vi "app - monitor RUS scan.vi"(10 "normalize phase":bool) -> ()   [LabVIEW 2015]
uses:
  complex region.ctl
  lorentzian.ctl
  circle corners.ctl
  cursor winow.ctl
  scale - offset gauge.ctl
  <vilib>/event_ctls.llb/eventvkey.ctl
  peak -- parameters -- complex fit.ctl
  wavepacket.ctl
  filter method control.ctl
  parameters -- scan monitor control.ctl
  monitor state.ctl
  peak monitor ctl - V2.ctl
  interpolation state - real.ctl
  countdown control.ctl
  cursor window action.ctl
  plot refs -- filter related.ctl
  monitor action.ctl
  read scan file control.ctl
  ctl -- name dispatcher -- action.ctl
  Q -- check range -- i -- real - window.vi
  array -- find interval - real.vi
  next chunk - read-write freq PID file - atomic actions .vi
  Q -- check range -- i -- integer.vi
  aggregator - vi - real - atomic.vi
  switch - C.vi
  acquire cursor window data.vi
  filter - complex - four.vi
  peak -- PM find lorenzian - V2.vi
  Q - not nan -- real.vi
  array -- find index - real.vi
  array -- interpolate -- i.vi
  Q - not nan -- integer.vi
  linear interpolation - real.vi
  tale of three indices.vi
  filter -- window span logic.vi
  linear interp iiii- complex - z-omega - divide.vi
  linear interpolation iiii- complex.vi
  containing bix.vi
  peak -- guess at omega -- dzdomega.vi
  command stack.vi
  tale of three indices -- check state.vi
  linear interp iiii- complex - z-omega.vi
  line -- complex.vi
  peak -- z center from mult phase points.vi
  peak -- estimate for lorentzian.vi
  peak -- fake phase around center.vi
  peak -- get weights.vi
  peak -- four corner circle transformation logic.vi
  peak - fit phase around center - V1.vi
  <vilib>/Analysis/baseanly.llb/A x B.vi
  <vilib>/Analysis/baseanly.llb/Complex A x B.vi
  circle center from three points.vi
  <vilib>/Utility/error.llb/Clear Errors.vi
  <vilib>/Utility/libraryn.llb/Check if File or Folder Exists.vi
  file -- read list of lines.vi
  parse -- find first line.vi
  parse -- get list of matches -- numbers.vi
  <vilib>/Utility/file.llb/Write To Spreadsheet File (string).vi
  <vilib>/gmath/function.llb/Binomial Coefficient.vi
  monitor -- write section files.vi
  <vilib>/Analysis/Matrix/Numeric/Conversions/Array To Matrix.vi
  <vilib>/Analysis/Matrix/Numeric/Conversions/Array To Matrix - RA2.vi
  <vilib>/Analysis/baseanly.llb/Inverse Matrix.vi
  <vilib>/Analysis/baseanly.llb/Real Inverse Matrix.vi
  array - generate range.vi
  peak -- fit function -- arctan.vi
  <vilib>/gmath/NumericalOptimization/Nonlinear Curve Fit.vi
  <vilib>/gmath/NumericalOptimization/Nonlinear Curve Fit LM.vi
  filter pipe - plot staff - more - V2.vi
panel:
  out "current resonance #":i32
  in  "overwriting !!":bool
  in  "current resonance #":i32
  in  "overwrite (d)":enum16{"DUMP", "WORK", ""}(ring)
  in  "Tab : monitor":enum32{"main", "EDIT"}(tab)=enum."EDIT"
  in  "scan monitor control":T1={"gamma acc. frac. - min "=0.3, "gamma acc frac.. - max"=3.0, "peak acc. fraction (af)"=5.0, "min peak acc. window (kHz)"=0.5, "use"=enum."fraction", "abs gamma min(kHz)"=0.005, "abs gamma max(kHz)"=5.0, "# points"=5, "gamma-factor (fa)"=5.0, "interpolate"=enum."line", "init"=TRUE, "Unique strike parameters"=TRUE, "max peak acc. window (kHz)"=10.0, "spacing factor"=1.5, "iterate #"=1, "overwrite ctl?"=FALSE, "write _m files?"=FALSE, "max slope (kHz/sweep)"=0.5, "funnel state"=enum."funnel open"}
  in  "monitor state":T2={"header - gamma"=[], "header - frequency"=[], "# of peaks"=32, "peaks OK"=FALSE}
  in  "autopilot":enum32{"on", "off"}(tab)=enum."off"
  in  "timer \"v\"":dbl(slide)=4.22200000169687 min=-2147482748.0000002 max=2129711151.0 step=0.01 scale=0.0..5.0 scale format="%#3_3f"
  in  "timer  \"update\"":dbl(slide)=9.242000002413988 min=-2147482714.9999983 max=2129711151.0 step=0.010000000000000002 scale=0.0..10.0 scale format="%#3_3f"
  in  "Temperature (K)":dbl=201.512
  in  "Magn Field (T)":dbl
  in  "Array of states":T3[](array[typedef])=[{"delta"=-0.0016575432837271364, "gamma"=0.76553, "exp"=652.9113, "found?"=TRUE, "found"=652.9096424567163, "gamma found"=0.7013829844109373, "init linear"=FALSE, "interpolate"=enum."line", "gamma-factor"=5.0, "slope"=-0.0044851701449078974, "update freq?"=TRUE, "update gamma?"=TRUE, "acc factor"=5.0, "linear interpolation state"={"requested size"=5, "Array"=[652.9241022479541, 652.9241022479541, 652.9081701289798, 652.9081701289798, 652.9096424567163], "actual number of elements"=5}, "ind"=0.0, "gamma ratio"=0.9162057455761854, "gamma off limit?"=FALSE, "freq off limit?"=FALSE}, {"delta"=0.003759118773814407, "gamma"=0.17466, "exp"=1036.47326, "found?"=TRUE, "found"=1036.4770191187738, "gamma found"=0.18203135700796666, "init linear"=FALSE, "interpolate"=enum."line", "gamma-factor"=5.0, "slope"=-0.0007907161774346605, "update freq?"=TRUE, "update gamma?"=TRUE, "acc factor"=5.0, "linear interpolation state"={"requested size"=5, "Array"=[1036.4789192628243, 1036.4789192628243, 1036.4748123891509, 1036.4748123891509, 1036.4770191187738], "actual number of elements"=5}, "ind"=1.0, "gamma ratio"=1.042204036459216, "gamma off limit?"=FALSE, "freq off limit?"=FALSE}, {"delta"=0.0049091040252733364, "gamma"=0.2876, "exp"=1456.4571, "found?"=TRUE, "found"=1456.4620091040254, "gamma found"=0.29018960202050387, "init linear"=FALSE, "interpolate"=enum."line", "gamma-factor"=5.0, "slope"=0.0005201884449343197, "update freq?"=TRUE, "update gamma?"=TRUE, "acc factor"=5.0, "linear interpolation state"={"requested size"=5, "Array"=[1456.4592147196108, 1456.4592147196108, 1456.4588278352328, 1456.4588278352328, 1456.4620091040254], "actual number of elements"=5}, "ind"=2.0, "gamma ratio"=1.0090041794871483, "gamma off limit?"=FALSE, "freq off limit?"=FALSE}, {"delta"=0.0007394967815343989, "gamma"=0.09637, "exp"=1508.93353, "found?"=TRUE, "found"=1508.9342694967816, "gamma found"=0.09651911838128847, "init linear"=FALSE, "interpolate"=enum."line", "gamma-factor"=5.0, "slope"=-0.00010129910398973152, "update freq?"=TRUE, "update gamma?"=TRUE, "acc factor"=5.0, "linear interpolation state"={"requested size"=5, "Array"=[1508.934330293854, 1508.934330293854, 1508.9334388969608, 1508.9334388969608, 1508.9342694967816], "actual number of elements"=5}, "ind"=3.0, "gamma ratio"=1.0015473527164935, "gamma off limit?"=FALSE, "freq off limit?"=FALSE}, {"delta"=-0.029278381005497067, "gamma"=0.50061, "exp"=1568.62295, "found?"=TRUE, "found"=1568.5936716189944, "gamma found"=0.29241762919205017, "init linear"=FALSE, "interpolate"=enum."line", "gamma-factor"=5.0, "slope"=0.002435031997738406, "update freq?"=TRUE, "update gamma?"=TRUE, "acc factor"=5.0, "linear interpolation state"={"requested size"=5, "Array"=[1568.5938152073131, 1568.5938152073131, 1568.618452703927, 1568.618452703927, 1568.5936716189944], "actual number of elements"=5}, "ind"=4.0, "gamma ratio"=0.5841226287769924, "gamma off limit?"=FALSE, "freq off limit?"=FALSE}, {"delta"=0.0026202347487469524, "gamma"=0.0806, "exp"=1635.60553, "found?"=TRUE, "found"=1635.6081502347488, "gamma found"=0.08233227541925552, "init linear"=FALSE, "interpolate"=enum."line", "gamma-factor"=5.0, "slope"=-0.0002922362121171318, "update freq?"=TRUE, "update gamma?"=TRUE, "acc factor"=5.0, "linear interpolation state"={"requested size"=5, "Array"=[1635.6087113801916, 1635.6087113801916, 1635.6069113089588, 1635.6069113089588, 1635.6081502347488], "actual number of elements"=5}, "ind"=5.0, "gamma ratio"=1.0214922508592494, "gamma off limit?"=FALSE, "freq off limit?"=FALSE}, {"delta"=-0.002563017279953783, "gamma"=0.23948, "exp"=1764.33943, "found?"=TRUE, "found"=1764.33686698272, "gamma found"=0.24236340731954384, "init linear"=FALSE, "interpolate"=enum."line", "gamma-factor"=5.0, "slope"=-0.0006999494679621421, "update freq?"=TRUE, "update gamma?"=TRUE, "acc factor"=5.0, "linear interpolation state"={"requested size"=5, "Array"=[1764.3399842040806, 1764.3399842040806, 1764.339219152121, 1764.339219152121, 1764.33686698272], "actual number of elements"=5}, "ind"=6.0, "gamma ratio"=1.012040284447736, "gamma off limit?"=FALSE, "freq off limit?"=FALSE}, {"delta"=0.0013207520305513754, "gamma"=0.09629, "exp"=2205.10687, "found?"=TRUE, "found"=2205.1081907520306, "gamma found"=0.0924387831546914, "init linear"=FALSE, "interpolate"=enum."line", "gamma-factor"=5.0, "slope"=-7.088923128321767e-05, "update freq?"=TRUE, "update gamma?"=TRUE, "acc factor"=5.0, "linear interpolation state"={"requested size"=5, "Array"=[2205.108115975172, 2205.108115975172, 2205.1072575291464, 2205.1072575291464, 2205.1081907520306], "actual number of elements"=5}, "ind"=7.0, "gamma ratio"=0.9600039791742797, "gamma off limit?"=FALSE, "freq off limit?"=FALSE}, {"delta"=0.003409232488138514, "gamma"=0.15471, "exp"=2247.57115, "found?"=TRUE, "found"=2247.5745592324884, "gamma found"=0.1527741784741036, "init linear"=FALSE, "interpolate"=enum."line", "gamma-factor"=5.0, "slope"=-0.0009672962635522708, "update freq?"=TRUE, "update gamma?"=TRUE, "acc factor"=5.0, "linear interpolation state"={"requested size"=5, "Array"=[2247.5776758034717, 2247.5776758034717, 2247.574235982803, 2247.574235982803, 2247.5745592324884], "actual number of elements"=5}, "ind"=8.0, "gamma ratio"=0.9874874182283214, "gamma off limit?"=FALSE, "freq off limit?"=FALSE}, {"delta"=-0.008548894449631916, "gamma"=0.16479, "exp"=2285.77663, "found?"=TRUE, "found"=2285.76808110555, "gamma found"=0.1267187147828005, "init linear"=FALSE, "interpolate"=enum."line", "gamma-factor"=5.0, "slope"=-0.0016395337344147264, "update freq?"=TRUE, "update gamma?"=TRUE, "acc factor"=5.0, "linear interpolation state"={"requested size"=5, "Array"=[2285.7766292086317, 2285.7766292086317, 2285.77733007745, 2285.77733007745, 2285.76808110555], "actual number of elements"=5}, "ind"=9.0, "gamma ratio"=0.7689709010425421, "gamma off limit?"=FALSE, "freq off limit?"=FALSE}, {"delta"=0.0004447395758688799, "gamma"=0.21964, "exp"=2405.10472, "found?"=TRUE, "found"=2405.1051647395757, "gamma found"=0.22044726667002684, "init linear"=FALSE, "interpolate"=enum."line", "gamma-factor"=5.0, "slope"=-0.0008384914183989168, "update freq?"=TRUE, "update gamma?"=TRUE, "acc factor"=5.0, "linear interpolation state"={"requested size"=5, "Array"=[2405.1081612139637, 2405.1081612139637, 2405.10576924856, 2405.10576924856, 2405.1051647395757], "actual number of elements"=5}, "ind"=10.0, "gamma ratio"=1.0036754082590915, "gamma off limit?"=FALSE, "freq off limit?"=FALSE}, {"delta"=0.0003001280488206248, "gamma"=0.22537, "exp"=2483.53635, "found?"=TRUE, "found"=2483.5366501280487, "gamma found"=0.2213622002178064, "init linear"=FALSE, "interpolate"=enum."line", "gamma-factor"=5.0, "slope"=-5.884840269573033e-05, "update freq?"=TRUE, "update gamma?"=TRUE, "acc factor"=5.0, "linear interpolation state"={"requested size"=5, "Array"=[2483.536882570466, 2483.536882570466, 2483.5367589712696, 2483.5367589712696, 2483.5366501280487], "actual number of elements"=5}, "ind"=11.0, "gamma ratio"=0.9822168000080153, "gamma off limit?"=FALSE, "freq off limit?"=FALSE}, {"delta"=-0.00047377254441016703, "gamma"=0.1374, "exp"=2613.48596, "found?"=TRUE, "found"=2613.4854862274556, "gamma found"=0.13919976502630776, "init linear"=FALSE, "interpolate"=enum."line", "gamma-factor"=5.0, "slope"=-0.0004374731567804702, "update freq?"=TRUE, "update gamma?"=TRUE, "acc factor"=5.0, "linear interpolation state"={"requested size"=5, "Array"=[2613.4871697330486, 2613.4871697330486, 2613.4861620126653, 2613.4861620126653, 2613.4854862274556], "actual number of elements"=5}, "ind"=12.0, "gamma ratio"=1.0130987265379023, "gamma off limit?"=FALSE, "freq off limit?"=FALSE}, {"delta"=-0.0014333203166643216, "gamma"=0.23275, "exp"=2775.83282, "found?"=TRUE, "found"=2775.8313866796834, "gamma found"=0.2800873248387451, "init linear"=FALSE, "interpolate"=enum."line", "gamma-factor"=5.0, "slope"=9.053546469658613e-05, "update freq?"=TRUE, "update gamma?"=TRUE, "acc factor"=5.0, "linear interpolation state"={"requested size"=5, "Array"=[2775.8316113301, 2775.8316113301, 2775.8329659855785, 2775.8329659855785, 2775.8313866796834], "actual number of elements"=5}, "ind"=13.0, "gamma ratio"=1.2033827060740927, "gamma off limit?"=FALSE, "freq off limit?"=FALSE}, {"delta"=0.001513914386578108, "gamma"=0.0716, "exp"=2886.62499, "found?"=TRUE, "found"=2886.6265039143864, "gamma found"=0.07112662438840253, "init linear"=FALSE, "interpolate"=enum."line", "gamma-factor"=5.0, "slope"=-0.0006266225839499384, "update freq?"=TRUE, "update gamma?"=TRUE, "acc factor"=5.0, "linear interpolation state"={"requested size"=5, "Array"=[2886.628416499212, 2886.628416499212, 2886.6259754430316, 2886.6259754430316, 2886.6265039143864], "actual number of elements"=5}, "ind"=14.0, "gamma ratio"=0.9933886087765718, "gamma off limit?"=FALSE, "freq off limit?"=FALSE}, {"delta"=0.006262894615701953, "gamma"=0.14682, "exp"=2925.52376, "found?"=TRUE, "found"=2925.5300228946157, "gamma found"=0.14212049264176846, "init linear"=FALSE, "interpolate"=enum."line", "gamma-factor"=5.0, "slope"=-0.0013607249583583326, "update freq?"=TRUE, "update gamma?"=TRUE, "acc factor"=5.0, "linear interpolation state"={"requested size"=5, "Array"=[2925.5337999193525, 2925.5337999193525, 2925.5277467192377, 2925.5277467192377, 2925.5300228946157], "actual number of elements"=5}, "ind"=15.0, "gamma ratio"=0.9679913679455691, "gamma off limit?"=FALSE, "freq off limit?"=FALSE}, {"delta"=0.0008407358172917156, "gamma"=0.05724, "exp"=2968.74884, "found?"=TRUE, "found"=2968.7496807358175, "gamma found"=0.056604877858379594, "init linear"=FALSE, "interpolate"=enum."line", "gamma-factor"=5.0, "slope"=6.453693960793316e-05, "update freq?"=TRUE, "update gamma?"=TRUE, "acc factor"=5.0, "linear interpolation state"={"requested size"=5, "Array"=[2968.7492258726284, 2968.7492258726284, 2968.7489615156423, 2968.7489615156423, 2968.7496807358175], "actual number of elements"=5}, "ind"=16.0, "gamma ratio"=0.9889042253385674, "gamma off limit?"=FALSE, "freq off limit?"=FALSE}, {"delta"=0.0004893467435067578, "gamma"=0.18507, "exp"=3117.27562, "found?"=TRUE, "found"=3117.2761093467434, "gamma found"=0.18508310581473786, "init linear"=FALSE, "interpolate"=enum."line", "gamma-factor"=5.0, "slope"=-0.000674382079159841, "update freq?"=TRUE, "update gamma?"=TRUE, "acc factor"=5.0, "linear interpolation state"={"requested size"=5, "Array"=[3117.278479994366, 3117.278479994366, 3117.27647746882, 3117.27647746882, 3117.2761093467434], "actual number of elements"=5}, "ind"=17.0, "gamma ratio"=1.0000708154467923, "gamma off limit?"=FALSE, "freq off limit?"=FALSE}, {"delta"=0.0009432243264200224, "gamma"=0.11467, "exp"=3141.4319, "found?"=TRUE, "found"=3141.4328432243265, "gamma found"=0.11506466086057514, "init linear"=FALSE, "interpolate"=enum."line", "gamma-factor"=5.0, "slope"=-0.0002722086093854159, "update freq?"=TRUE, "update gamma?"=TRUE, "acc factor"=5.0, "linear interpolation state"={"requested size"=5, "Array"=[3141.4337316093643, 3141.4337316093643, 3141.432786293347, 3141.432786293347, 3141.4328432243265], "actual number of elements"=5}, "ind"=18.0, "gamma ratio"=1.0034417097808943, "gamma off limit?"=FALSE, "freq off limit?"=FALSE}, {"delta"=0.006890674223541282, "gamma"=0.19401, "exp"=3268.65403, "found?"=TRUE, "found"=3268.6609206742237, "gamma found"=0.1947000973954296, "init linear"=FALSE, "interpolate"=enum."line", "gamma-factor"=5.0, "slope"=0.001370561413350515, "update freq?"=TRUE, "update gamma?"=TRUE, "acc factor"=5.0, "linear interpolation state"={"requested size"=5, "Array"=[3268.654487682439, 3268.654487682439, 3268.6553273130035, 3268.6553273130035, 3268.6609206742237], "actual number of elements"=5}, "ind"=19.0, "gamma ratio"=1.0035570197176928, "gamma off limit?"=FALSE, "freq off limit?"=FALSE}, {"delta"=-0.00036122355459156097, "gamma"=0.09375, "exp"=3447.74234, "found?"=TRUE, "found"=3447.741978776445, "gamma found"=0.09343849466512388, "init linear"=FALSE, "interpolate"=enum."line", "gamma-factor"=5.0, "slope"=-0.0002539216459263116, "update freq?"=TRUE, "update gamma?"=TRUE, "acc factor"=5.0, "linear interpolation state"={"requested size"=5, "Array"=[3447.7428802682552, 3447.7428802682552, 3447.742144035429, 3447.742144035429, 3447.741978776445], "actual number of elements"=5}, "ind"=20.0, "gamma ratio"=0.9966772764279881, "gamma off limit?"=FALSE, "freq off limit?"=FALSE}, {"delta"=-3486.5123, "gamma"=0.01485, "exp"=3486.5123, "found?"=FALSE, "found"=0.0, "gamma found"=0.0, "init linear"=TRUE, "interpolate"=enum."line", "gamma-factor"=5.0, "slope"=0.0, "update freq?"=FALSE, "update gamma?"=FALSE, "acc factor"=5.0, "linear interpolation state"={"requested size"=5, "Array"=[0.0, 0.0, 0.0, 0.0, 3486.5122984940626], "actual number of elements"=1}, "ind"=21.0, "gamma ratio"=0.0, "gamma off limit?"=TRUE, "freq off limit?"=TRUE}, {"delta"=0.005188108485072007, "gamma"=0.2862, "exp"=3737.75053, "found?"=TRUE, "found"=3737.755718108485, "gamma found"=0.25947921890028686, "init linear"=FALSE, "interpolate"=enum."line", "gamma-factor"=5.0, "slope"=-0.0006564744841307402, "update freq?"=TRUE, "update gamma?"=TRUE, "acc factor"=5.0, "linear interpolation state"={"requested size"=5, "Array"=[3737.7568178710067, 3737.7568178710067, 3737.752452651206, 3737.752452651206, 3737.755718108485], "actual number of elements"=5}, "ind"=22.0, "gamma ratio"=0.9066359849765439, "gamma off limit?"=FALSE, "freq off limit?"=FALSE}, {"delta"=0.05791749378431632, "gamma"=0.1209, "exp"=3773.78708, "found?"=FALSE, "found"=3773.8449974937844, "gamma found"=0.0018969298658040622, "init linear"=FALSE, "interpolate"=enum."line", "gamma-factor"=7.0, "slope"=-0.027493364620750072, "update freq?"=TRUE, "update gamma?"=TRUE, "acc factor"=7.0, "linear interpolation state"={"requested size"=5, "Array"=[0.0, 3773.880271706499, 3773.8206547185614, 3773.825284977259, 3773.7870837381997], "actual number of elements"=4}, "ind"=23.0, "gamma ratio"=0.015690073331712674, "gamma off limit?"=TRUE, "freq off limit?"=FALSE}, {"delta"=0.0016448427732029813, "gamma"=0.14541, "exp"=4176.53307, "found?"=TRUE, "found"=4176.534714842774, "gamma found"=0.14055145401454877, "init linear"=FALSE, "interpolate"=enum."line", "gamma-factor"=5.0, "slope"=0.001082140458165668, "update freq?"=TRUE, "update gamma?"=TRUE, "acc factor"=5.0, "linear interpolation state"={"requested size"=5, "Array"=[4176.530918624351, 4176.530918624351, 4176.534147592093, 4176.534147592093, 4176.534714842774], "actual number of elements"=5}, "ind"=24.0, "gamma ratio"=0.9665872636995307, "gamma off limit?"=FALSE, "freq off limit?"=FALSE}, {"delta"=0.006093070963288483, "gamma"=0.07631, "exp"=4238.40966, "found?"=TRUE, "found"=4238.415753070964, "gamma found"=0.07370934433890397, "init linear"=FALSE, "interpolate"=enum."line", "gamma-factor"=5.0, "slope"=-0.0001927513594273478, "update freq?"=TRUE, "update gamma?"=TRUE, "acc factor"=5.0, "linear interpolation state"={"requested size"=5, "Array"=[4238.415194475135, 4238.415194475135, 4238.412149769886, 4238.412149769886, 4238.415753070964], "actual number of elements"=5}, "ind"=25.0, "gamma ratio"=0.9659198576713925, "gamma off limit?"=FALSE, "freq off limit?"=FALSE}, {"delta"=0.0014712240090375417, "gamma"=0.10797, "exp"=4931.57573, "found?"=TRUE, "found"=4931.577201224009, "gamma found"=0.1106825599113035, "init linear"=FALSE, "interpolate"=enum."line", "gamma-factor"=5.0, "slope"=0.0010064907773630694, "update freq?"=TRUE, "update gamma?"=TRUE, "acc factor"=5.0, "linear interpolation state"={"requested size"=5, "Array"=[4931.573629158262, 4931.573629158262, 4931.5765499345425, 4931.5765499345425, 4931.577201224009], "actual number of elements"=5}, "ind"=26.0, "gamma ratio"=1.0251232741622998, "gamma off limit?"=FALSE, "freq off limit?"=FALSE}, {"delta"=0.01094153662052122, "gamma"=0.05188, "exp"=5475.82656, "found?"=TRUE, "found"=5475.837501536621, "gamma found"=0.11863591544266465, "init linear"=FALSE, "interpolate"=enum."line", "gamma-factor"=8.0, "slope"=0.0012847163761034609, "update freq?"=TRUE, "update gamma?"=TRUE, "acc factor"=8.0, "linear interpolation state"={"requested size"=5, "Array"=[5475.831455900791, 5475.831455900791, 5475.832211792886, 5475.832211792886, 5475.837501536621], "actual number of elements"=5}, "ind"=27.0, "gamma ratio"=2.2867369977383314, "gamma off limit?"=FALSE, "freq off limit?"=FALSE}, {"delta"=-5768.35916, "gamma"=0.005, "exp"=5768.35916, "found?"=FALSE, "found"=0.0, "gamma found"=0.0, "init linear"=TRUE, "interpolate"=enum."line", "gamma-factor"=5.0, "slope"=0.0, "update freq?"=FALSE, "update gamma?"=FALSE, "acc factor"=5.0, "linear interpolation state"={"requested size"=5, "Array"=[0.0, 0.0, 0.0, 0.0, 5768.359158074293], "actual number of elements"=1}, "ind"=28.0, "gamma ratio"=0.0, "gamma off limit?"=TRUE, "freq off limit?"=TRUE}, {"delta"=18.256138418231785, "gamma"=0.02905, "exp"=6148.70194, "found?"=FALSE, "found"=6166.958078418232, "gamma found"=4.5314912463139816e-05, "init linear"=TRUE, "interpolate"=enum."line", "gamma-factor"=5.0, "slope"=0.0, "update freq?"=FALSE, "update gamma?"=FALSE, "acc factor"=5.0, "linear interpolation state"={"requested size"=5, "Array"=[0.0, 0.0, 0.0, 0.0, 6148.701943422434], "actual number of elements"=1}, "ind"=29.0, "gamma ratio"=0.001559893716459202, "gamma off limit?"=TRUE, "freq off limit?"=TRUE}, {"delta"=0.004358224254247034, "gamma"=0.0424, "exp"=5751.24344, "found?"=TRUE, "found"=5751.247798224254, "gamma found"=0.0686871247901866, "init linear"=TRUE, "interpolate"=enum."line", "gamma-factor"=7.0, "slope"=0.0, "update freq?"=FALSE, "update gamma?"=FALSE, "acc factor"=7.0, "linear interpolation state"={"requested size"=5, "Array"=[0.0, 0.0, 0.0, 0.0, 5751.24344], "actual number of elements"=1}, "ind"=30.0, "gamma ratio"=1.619979358259118, "gamma off limit?"=FALSE, "freq off limit?"=FALSE}, {"delta"=0.02459476473813993, "gamma"=0.14229, "exp"=6300.95565, "found?"=TRUE, "found"=6300.980244764738, "gamma found"=0.1593322314931949, "init linear"=FALSE, "interpolate"=enum."line", "gamma-factor"=7.0, "slope"=0.001076212803600356, "update freq?"=TRUE, "update gamma?"=TRUE, "acc factor"=7.0, "linear interpolation state"={"requested size"=5, "Array"=[6300.9711810739645, 6300.9711810739645, 6300.963815820454, 6300.963815820454, 6300.980244764738], "actual number of elements"=5}, "ind"=31.0, "gamma ratio"=1.1197711117660756, "gamma off limit?"=FALSE, "freq off limit?"=FALSE}]
  in  "dump/work NEW (\"n\")":enum16{"DUMP", "WORK", ""}(ring)
  in  "NEW freq":dbl[](array[numeric])=[652.901381931682, 1036.4745243360126, 1456.4611794080774, 1508.93365767837, 1568.6109465842878, 1635.607002413974, 1764.33695489062, 2205.1075748844396, 2247.5727746722177, 2285.770281334339, 2405.104089658669, 2483.536610097096, 2613.485117524306, 2775.8323798686024, 2886.625177692022, 2925.5265410594843, 2968.74940471329, 3117.275181708386, 3141.432359180121, 3268.6602218172616, 3447.7416437118245, 3486.5122984940626, 3737.7528824071287, 3773.7595903735782, 4176.536215876507, 4238.4135100581225, 4931.5785313542565, 5475.8368215339215, 5768.359158074293, 6148.701943422434, 5751.24344, 6300.973276349126]
  in  "NEW gamma":dbl[](array[numeric])=[0.7013829844109373, 0.18203135700796666, 0.29018960202050387, 0.09651911838128847, 0.29241762919205017, 0.08233227541925552, 0.24236340731954384, 0.0924387831546914, 0.1527741784741036, 0.1267187147828005, 0.22044726667002684, 0.2213622002178064, 0.13919976502630776, 0.2800873248387451, 0.07112662438840253, 0.14212049264176846, 0.056604877858379594, 0.18508310581473786, 0.11506466086057514, 0.1947000973954296, 0.09343849466512388, 0.01485, 0.25947921890028686, 0.1209, 0.14055145401454877, 0.07370934433890397, 0.1106825599113035, 0.11863591544266465, 0.005, 0.02905, 0.0424, 0.1593322314931949]
  in  "OLD gamma":dbl[](array[numeric])
  in  "OLD freq":dbl[](array[numeric])
  out "cp lorentzian":T5={"Amplitude"=0.017781649209978104, "omega(0)"=653.3752688609701, "Gamma"=64.36082364251368, "phase"=2.362044339201428, "Q"=10.151754310822424, "Norm  Ampl"=nan, "z (inf)"=0.02262747381101565+0.008890453242250202i, "4corners"={"z (-pi/2)"=0.022625188172095752+0.009281166377616138i, "z(inf)"=0.02262747381101565+0.008890453242250202i, "z (pi/2)"=0.023018186946381587+0.008892738881170098i, "z center"=0.02282168755923867+0.009086952629393118i, "z(0)"=0.02301590130746169+0.009283452016536034i, "radius"=0.0002762806347654071}} {"z (inf)" format="%#9_9f"; "Q" format="%#9_9f"; "phase" format="%#9_9f"; "Gamma" format="%#9_9f"; "omega(0)" format="%#9_9f"}
  out "index":i32[](array[numeric])=[0, 1, 2, 3, 4, 5, 6, 7, 8, 9, 10, 11, 12, 13, 14, 15, 16, 17, 18, 19, 20, 21, 22, 23, 24, 25, 26, 27, 28, 29, 30, 31, 32, 33, 34, 35, 36, 37, 38, 39, 40, 41, 42, 43, 44, 45, 46, 47, 48, 49, 50, 51, 52, 53, 54, 55, 56, 57, 58, 59, 60, 61, 62, 63, 64, 65, 66, 67, 68, 69, 70, 71, 72, 73, 74, 75, 76, 77, 78, 79, 80, 81, 82, 83, 84, 85, 86, 87, 88, 89, 90, 91, 92, 93, 94, 95, 96, 97, 98, 99]
  in  "Tab : everything":T7(tab)
  in  "Tab :  Fit controls":enum32{"complex plane", "complex plane 2"}(tab)
  in  "Plot: fragment - filter":cluster{dbl[], dbl[]}[](graph)
  in  "scale gauge: Plot: complex plane - filter":dbl(slide)=0.00996 min=0.0 max=0.3 step=1e-05 scale=0.0001..0.3 scale format="%#_2g"
  in  "Plot: complex plane - filter":cluster{dbl[], dbl[]}[](graph)=[{array[252 elements], array[252 elements]}, {array[252 elements], array[252 elements]}, {[0.02330588676949013, 0.023305318955812702, 0.023303617755681592, 0.02330078988295652, 0.02329684649795919, 0.023291803163428635, 0.02328567978310216, 0.023278500523164408, 0.023270293716874463, 0.023261091752747418, 0.023250930946731706, 0.023239851398886638, 0.023227896835125793, 0.02321511443465082, 0.023201554643756665, 0.023187270976743113, 0.02317231980471828, 0.023156760133127598, 0.023140653368886308, 0.02312406307803438, 0.023107054734870437, 0.023089695463554563, 0.023072053773199947, 0.023054199287498703, 0.023036202469948946, 0.02301813434576759, 0.023000066221586235, 0.02298206940403648, 0.022964214918335234, 0.02294657322798062, 0.022929213956664744, 0.0229122056135008, 0.022895615322648874, 0.022879508558407584, 0.022863948886816903, 0.02284899771479207, 0.022834714047778516, 0.02282115425688436, 0.02280837185640939, 0.022796417292648544, 0.022785337744803475, 0.022775176938787764, 0.022765974974660718, 0.022757768168370773, 0.022750588908433022, 0.022744465528106547, 0.02273942219357599, 0.022735478808578662, 0.02273265093585359, 0.02273094973572248, 0.022730381922045052, 0.02273094973572248, 0.02273265093585359, 0.022735478808578662, 0.02273942219357599, 0.022744465528106547, 0.022750588908433022, 0.022757768168370773, 0.022765974974660718, 0.022775176938787764, 0.022785337744803475, 0.022796417292648544, 0.02280837185640939, 0.02282115425688436, 0.022834714047778516, 0.02284899771479207, 0.022863948886816903, 0.022879508558407584, 0.022895615322648877, 0.0229122056135008, 0.022929213956664744, 0.02294657322798062, 0.022964214918335234, 0.02298206940403648, 0.023000066221586235, 0.02301813434576759, 0.023036202469948946, 0.023054199287498703, 0.023072053773199947, 0.023089695463554563, 0.023107054734870437, 0.02312406307803438, 0.023140653368886304, 0.023156760133127598, 0.02317231980471828, 0.023187270976743113, 0.023201554643756665, 0.02321511443465082, 0.023227896835125793, 0.023239851398886638, 0.023250930946731706, 0.023261091752747418, 0.023270293716874463, 0.023278500523164408, 0.02328567978310216, 0.023291803163428635, 0.02329684649795919, 0.02330078988295652, 0.023303617755681592, 0.023305318955812702], [0.009264160688823775, 0.009282228813005132, 0.009300225630554887, 0.009318080116256133, 0.009335721806610747, 0.00935308107792662, 0.009370089421090565, 0.00938667971194249, 0.009402786476183781, 0.00941834614777446, 0.009433297319799297, 0.00944758098681285, 0.009461140777707005, 0.009473923178181978, 0.00948587774194282, 0.009496957289787888, 0.009507118095803603, 0.009516320059930647, 0.009524526866220592, 0.009531706126158343, 0.009537829506484819, 0.009542872841015376, 0.009546816226012703, 0.009549644098737778, 0.009551345298868886, 0.009551913112546313, 0.009551345298868886, 0.009549644098737778, 0.009546816226012703, 0.009542872841015376, 0.009537829506484819, 0.009531706126158343, 0.009524526866220592, 0.009516320059930647, 0.009507118095803603, 0.009496957289787888, 0.00948587774194282, 0.009473923178181978, 0.009461140777707005, 0.00944758098681285, 0.009433297319799297, 0.00941834614777446, 0.009402786476183781, 0.00938667971194249, 0.009370089421090565, 0.00935308107792662, 0.009335721806610747, 0.009318080116256133, 0.009300225630554887, 0.009282228813005132, 0.009264160688823775, 0.009246092564642417, 0.009228095747092662, 0.009210241261391416, 0.009192599571036802, 0.00917524029972093, 0.009158231956556982, 0.00914164166570506, 0.009125534901463768, 0.009109975229873089, 0.009095024057848252, 0.009080740390834698, 0.009067180599940544, 0.00905439819946557, 0.00904244363570473, 0.00903136408785966, 0.009021203281843946, 0.009012001317716902, 0.009003794511426957, 0.008996615251489206, 0.00899049187116273, 0.008985448536632173, 0.008981505151634846, 0.008978677278909771, 0.008976976078778664, 0.008976408265101236, 0.008976976078778664, 0.008978677278909771, 0.008981505151634846, 0.008985448536632173, 0.00899049187116273, 0.008996615251489206, 0.009003794511426957, 0.009012001317716902, 0.009021203281843946, 0.00903136408785966, 0.00904244363570473, 0.00905439819946557, 0.009067180599940544, 0.009080740390834698, 0.009095024057848252, 0.009109975229873089, 0.009125534901463768, 0.00914164166570506, 0.009158231956556984, 0.00917524029972093, 0.009192599571036804, 0.009210241261391416, 0.009228095747092662, 0.009246092564642417]}, {[-7.134950150070041e-05, 3.845143540140428e-06, 3.702069766946953e-05], [0.0001830739588743243, -6.1760698272413095e-06, -3.90775167372244e-06]}, {[-3.448933898232793e-05, -3.695183869243852e-05, -3.941433840254912e-05, -4.1876838112659715e-05, -4.433933782277031e-05, -4.680183753288091e-05, -4.926433724299151e-05, -5.1726836953102105e-05, -5.41893366632127e-05, -5.66518363733233e-05, -5.911433608343389e-05, -6.157683579354449e-05, -6.403933550365509e-05, -6.65018352137657e-05, -6.896433492387628e-05, -7.142683463398687e-05, -7.388933434409748e-05, -7.635183405420808e-05, -7.881433376431867e-05, -8.127683347442926e-05], [3.604811685728011e-05, 3.82835879236857e-05, 4.051905899009129e-05, 4.275453005649688e-05, 4.499000112290247e-05, 4.722547218930806e-05, 4.9460943255713647e-05, 5.169641432211924e-05, 5.393188538852483e-05, 5.616735645493042e-05, 5.840282752133601e-05, 6.063829858774159e-05, 6.287376965414718e-05, 6.510924072055277e-05, 6.734471178695836e-05, 6.958018285336396e-05, 7.181565391976955e-05, 7.405112498617514e-05, 7.628659605258073e-05, 7.852206711898632e-05]}, {[3.845143540140428e-06, 8.708015624839466e-06, 1.3570887709538504e-05, 1.843375979423754e-05, 2.329663187893658e-05, 2.815950396363562e-05, 3.302237604833465e-05, 3.788524813303369e-05, 4.274812021773273e-05, 4.761099230243177e-05, 5.247386438713081e-05, 5.7336736471829845e-05, 6.219960855652888e-05, 6.706248064122792e-05, 7.192535272592696e-05, 7.6788224810626e-05, 8.165109689532504e-05, 8.651396898002407e-05, 9.137684106472312e-05, 9.623971314942215e-05], [-6.1760698272413095e-06, -6.1760698272413095e-06, -6.1760698272413095e-06, -6.1760698272413095e-06, -6.1760698272413095e-06, -6.1760698272413095e-06, -6.1760698272413095e-06, -6.1760698272413095e-06, -6.1760698272413095e-06, -6.1760698272413095e-06, -6.1760698272413095e-06, -6.1760698272413095e-06, -6.1760698272413095e-06, -6.1760698272413095e-06, -6.1760698272413095e-06, -6.1760698272413095e-06, -6.1760698272413095e-06, -6.1760698272413095e-06, -6.1760698272413095e-06, -6.1760698272413095e-06]}]
  out "Plot: dz/domega":cluster{"omega out":dbl[], dbl[]}(graph)
  out "Plot: win omega":T8(graph)
  out "Plot: phase":cluster{"omega out":dbl[], dbl[]}(graph)
  out "Plot: phase around center":cluster{dbl[], dbl[]}[](graph)
  out "Plot: fragment":cluster{dbl[], dbl[]}[](graph)
  out "Plot: complex plane":cluster{dbl[], dbl[]}[](graph)=[{array[252 elements], array[252 elements]}, {[0.023097968194004077, 0.023095789638677925, 0.023089288329818373, 0.023078566796949824, 0.023063794125050354, 0.02304520328798058, 0.023023087474346726, 0.022997795463741137, 0.02296972612627978, 0.022939322132182232, 0.02290706297059788, 0.02287345738777559, 0.02283903536383148, 0.02280433975464586, 0.02276991773070175, 0.02273631214787946, 0.022704052986295107, 0.022673648992197558, 0.022645579654736202, 0.022620287644130613, 0.02259817183049676, 0.022579580993426985, 0.022564808321527515, 0.022554086788658965, 0.022547585479799414, 0.022545406924473262, 0.022547585479799414, 0.022554086788658965, 0.022564808321527515, 0.022579580993426985, 0.02259817183049676, 0.022620287644130613, 0.022645579654736202, 0.022673648992197558, 0.022704052986295107, 0.02273631214787946, 0.02276991773070175, 0.02280433975464586, 0.02283903536383148, 0.02287345738777559, 0.02290706297059788, 0.022939322132182232, 0.02296972612627978, 0.022997795463741137, 0.023023087474346726, 0.02304520328798058, 0.023063794125050354, 0.023078566796949824, 0.023089288329818373, 0.023095789638677925], [0.009086952629393118, 0.009121579774719465, 0.009155660829278761, 0.009188658314481572, 0.009220051840274506, 0.009249346312002228, 0.009276079738345919, 0.009299830517202365, 0.009320224084600974, 0.009336938821801342, 0.00934971112741292, 0.009358339574546407, 0.009362688087436124, 0.009362688087436124, 0.009358339574546407, 0.00934971112741292, 0.009336938821801342, 0.009320224084600974, 0.009299830517202365, 0.009276079738345919, 0.009249346312002228, 0.009220051840274506, 0.009188658314481572, 0.009155660829278761, 0.009121579774719465, 0.009086952629393118, 0.009052325484066771, 0.009018244429507475, 0.008985246944304663, 0.008953853418511728, 0.008924558946784008, 0.008897825520440317, 0.00887407474158387, 0.008853681174185262, 0.008836966436984894, 0.008824194131373315, 0.008815565684239829, 0.008811217171350113, 0.008811217171350113, 0.008815565684239829, 0.008824194131373315, 0.008836966436984894, 0.008853681174185262, 0.008874074741583872, 0.008897825520440317, 0.008924558946784008, 0.00895385341851173, 0.008985246944304665, 0.009018244429507475, 0.009052325484066771]}, {[0.02262747381101565, 0.02264689518583795, 0.022666316560660253, 0.022685737935482557, 0.022705159310304857, 0.022724580685127158, 0.02274400205994946, 0.022763423434771765, 0.022782844809594065, 0.022802266184416366, 0.02282168755923867, 0.022841108934060973, 0.022860530308883274, 0.022879951683705574, 0.022899373058527878, 0.02291879443335018, 0.02293821580817248, 0.022957637182994782, 0.022977058557817086, 0.02299647993263939], [0.008890453242250202, 0.008910103180964494, 0.008929753119678785, 0.008949403058393077, 0.008969052997107369, 0.008988702935821661, 0.009008352874535951, 0.009028002813250243, 0.009047652751964536, 0.009067302690678826, 0.009086952629393118, 0.00910660256810741, 0.0091262525068217, 0.009145902445535993, 0.009165552384250285, 0.009185202322964575, 0.009204852261678867, 0.00922450220039316, 0.009244152139107452, 0.009263802077821742]}, {[0.022625188172095752, 0.022644838110810042, 0.022664488049524336, 0.022684137988238626, 0.02270378792695292, 0.02272343786566721, 0.0227430878043815, 0.022762737743095795, 0.022782387681810085, 0.02280203762052438, 0.02282168755923867, 0.02284133749795296, 0.022860987436667254, 0.022880637375381544, 0.022900287314095838, 0.02291993725281013, 0.02293958719152442, 0.022959237130238713, 0.022978887068953003, 0.022998537007667297], [0.009281166377616138, 0.009261745002793836, 0.009242323627971534, 0.009222902253149232, 0.00920348087832693, 0.009184059503504628, 0.009164638128682326, 0.009145216753860024, 0.009125795379037722, 0.00910637400421542, 0.009086952629393118, 0.009067531254570816, 0.009048109879748514, 0.009028688504926212, 0.00900926713010391, 0.008989845755281608, 0.008970424380459306, 0.008951003005637004, 0.008931581630814702, 0.0089121602559924]}, {[0.07261837532525764, 0.06942766670373372, 0.066207951232092, 0.06296124112769602, 0.05968956547867602, 0.05639496897581505, 0.053079510634683594, 0.04974526250882208, 0.04639430839477468, 0.04302874252978439, 0.039650668282963, 0.03626219684075362, 0.03286544588750821, 0.029462538282003486, 0.026055600730723445, 0.022646762458737087, 0.019238153879001865, 0.01583190526092518, 0.012430145399015121, 0.009035000282453286], [0.1362918938354443, 0.13749217464602775, 0.1386123209817326, 0.13965163278756135, 0.14060946052746642, 0.14148520559028904, 0.14227832066387164, 0.14298831007711024, 0.14361473010973275, 0.1441571892696096, 0.1446153485374237, 0.14498892157854637, 0.14527767492198723, 0.14548142810630602, 0.14560005379239493, 0.1456334778430616, 0.1455816793693624, 0.1454446907436572, 0.14522259757937797, 0.1449155386775229]}, {[0.07989364128996873, 0.0762349620706213, 0.0725430216631388, 0.06882012741009808, 0.06506860599922182, 0.061290802009274566, 0.05748907644477715, 0.05366580526045595, 0.049823377876348274, 0.04596419568449275, 0.042090670548137546, 0.03820522329440413, 0.034310282201349386, 0.03040828148037064, 0.02650165975490286, 0.0225928585363585, 0.018684320698262112, 0.014778488949534183, 0.010877804307877315, 0.0069847045742197425], [0.1549217222067073, 0.156298044202843, 0.15758247866778458, 0.1587742228718015, 0.15987253201355936, 0.16087671968559594, 0.161786158303304, 0.16260027949715092, 0.1633185744678914, 0.16394059430455019, 0.164465950264977, 0.16489431401879767, 0.16522541785260988, 0.16545905483729542, 0.16559507895734402, 0.16563340520210848, 0.16557400961893337, 0.16541692932812477, 0.16516226249975124, 0.16481016829229078]}, {array[252 elements], array[252 elements]}]
  in  "scale gauge: Plot: complex plane":dbl(slide)=0.0009400000000000001 min=0.0 max=0.3 step=1e-05 scale=0.0001..0.3 scale format="%#_2g"
  in  "plot staff":enum16{"plot", "do not plot", "a"}(ring)=enum."do not plot"
  out "pm lorentzian":T5={"Amplitude"=0.017781649209978104, "omega(0)"=653.3752688609701, "Gamma"=64.36082364251368, "phase"=2.362044339201428, "Q"=10.151754310822424, "Norm  Ampl"=nan, "z (inf)"=0.02262747381101565+0.008890453242250202i, "4corners"={"z (-pi/2)"=0.022625188172095752+0.009281166377616138i, "z(inf)"=0.02262747381101565+0.008890453242250202i, "z (pi/2)"=0.023018186946381587+0.008892738881170098i, "z center"=0.02282168755923867+0.009086952629393118i, "z(0)"=0.02301590130746169+0.009283452016536034i, "radius"=0.0002762806347654071}} {"z (inf)" format="%#9_9f"; "Q" format="%#9_9f"; "phase" format="%#9_9f"; "Gamma" format="%#9_9f"; "omega(0)" format="%#9_9f"}
  in  "use fast fit?":bool
  out "window width (kHz)":dbl=14.596141892560372
  out "window center (kHz)":dbl=652.9113
  out "# of points in window":dbl=251.65761883724736
  in  "Tab : all plot":enum32{"Page 1"}(tab)
  in  "scale gauge : All plot":T9={"scale offset"=0.5005000000000001, "scale range"=0.019950000000000002} {"scale range" min=0.0 max=1.0 step=1e-05 scale=0.001..1.0 scale format="%#_2g"; "scale offset" min=0.0 max=1.0 step=1e-05 scale=0.001..1.0 scale format="%#_2g"}
  out "Plot: All":cluster{"all rows":dbl[], "all rows":dbl[]}[](graph)
  in  "Sweep folder path":path=path "D:/Technique/RUS/RTe3/LaTe3_FisherXX27/7_test"
  out "scan file found":bool=TRUE
  in  "source":enum16{"last scan file", "manual"}(ring)
  out "complex region":T10={"max re"=1.5, "min re"=-1.5, "max im"=1.5, "min im"=-1.5, "delta re"=3.0, "delta im"=3.0, "center re"=0.0, "delta  z"=3.0+3.0i, "center im"=0.0, "center z"=0.0+0.0i, "d im"=0.0, "d re"=0.0, "d z"=0.0+0.0i}
  in  "cursor bracket: All, data window":T11={"left"=645.6132290537198, "right "=660.2093709462802, "center"=652.9113, "window"=14.596141892560372, "cursors"=[0, 1, 2], "relative"=1, "absolute"=1, "fixed vertical offset"=0.0, "vertical offset"=0.0, "skew"=0.0, "default window frac"=0.1, "kind"=enum."symmetric", "skew.left"=0.5, "skew.right"=0.5, "Plot ref"=refnum, "wing order"=enum."forw"}
  out "all:min omega":dbl=100.0
  out "all:max omega":dbl=2999.884
  in  "file path":path=path "D:/Technique/RUS/RTe3/LaTe3_FisherXX27/7_test/November_2015/111915/201.51200K_100_3000_2.00000V_0.00000T_Nov19-2015__12-01-52_001_111915.bin"
  in  "Tab : parameters":enum32{"Page 1"}(tab)
  out "VKey":T12
  out "Char":i16=82
  in  "parameters: complex fit":T13={"main VI path"=path "E:/ProjectLocker/LANL/Libraries/control rus sweep -- library/monitor RUS scan.vi", "scale factor"=3.0, "# of grid points"=150, "parameters: wavepacket"={"R"=0.5, "wave number"=22.0, "delta k"=7.0, "radii vector"=[], "radial section"=[], "wave vector"=22.0, "wavepacket is"=TRUE}, "span"=0.33799, "interference ?"=enum."pm zcenter", "filter method"=enum."three"} {"span" min=0.0 max=0.5 step=1e-05 scale=0.0001..0.5 scale format="%#_5f"; "parameters: wavepacket"."delta k" format="%#_3f"; "parameters: wavepacket"."wave number" format="%#_3f"; "parameters: wavepacket"."R" format="%#_3f"}
  out "4corners":T6={"z (-pi/2)"=nan+nani, "z(inf)"=nan+nani, "z (pi/2)"=nan+nani, "z center"=nan+nani, "z(0)"=nan+nani, "radius"=nan}
  out "good lorentzian":T5={"Amplitude"=0.017781649209978104, "omega(0)"=653.3752688609701, "Gamma"=64.36082364251368, "phase"=2.362044339201428, "Q"=10.151754310822424, "Norm  Ampl"=nan, "z (inf)"=0.02262747381101565+0.008890453242250202i, "4corners"={"z (-pi/2)"=0.022625188172095752+0.009281166377616138i, "z(inf)"=0.02262747381101565+0.008890453242250202i, "z (pi/2)"=0.023018186946381587+0.008892738881170098i, "z center"=0.02282168755923867+0.009086952629393118i, "z(0)"=0.02301590130746169+0.009283452016536034i, "radius"=0.0002762806347654071}} {"z (inf)" format="%#9_9f"; "Q" format="%#9_9f"; "phase" format="%#9_9f"; "Gamma" format="%#9_9f"; "omega(0)" format="%#9_9f"}
  # "three strikes"
  # "search window"
  # "linear extrapolation"
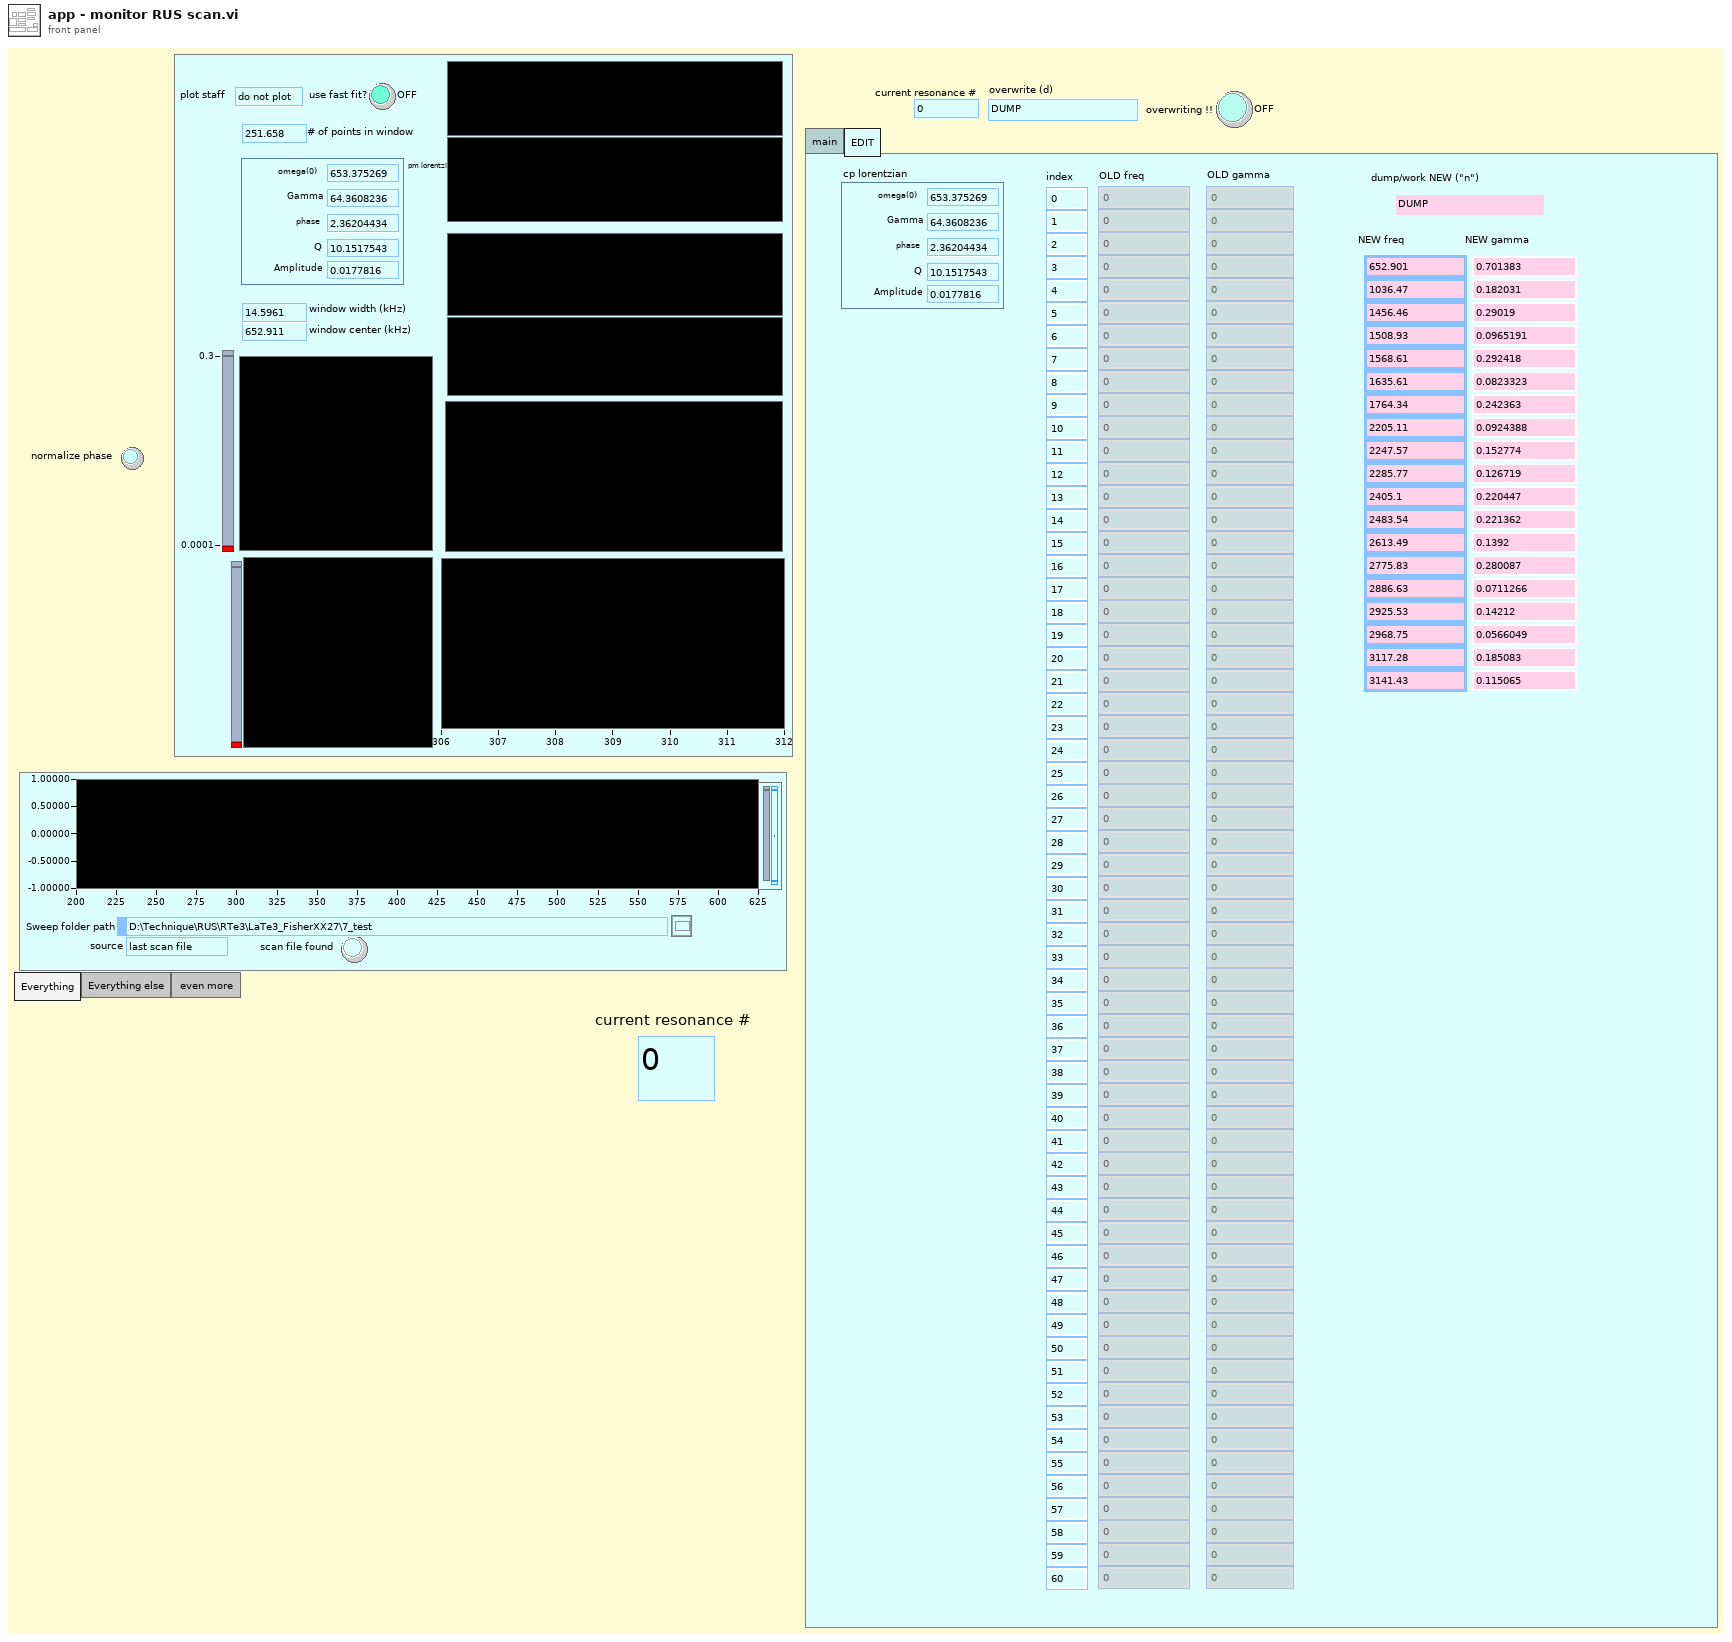
[diagram p1: front panel]
types:
  T1 = typedef "parameters -- scan monitor control.ctl" = cluster{"gamma acc. frac. - min ":dbl, "gamma acc frac.. - max":dbl, "peak acc. fraction (af)":dbl, "min peak acc. window (kHz)":dbl, "use":enum16{"window", "fraction"}, "abs gamma min(kHz)":dbl, "abs gamma max(kHz)":dbl, "# points":i32, "gamma-factor (fa)":dbl, "interpolate":enum16{"line", "last"}, "init":bool, "Unique strike parameters":bool, "max peak acc. window (kHz)":dbl, "spacing factor":dbl, "iterate #":i32, "overwrite ctl?":bool, "write _m files?":bool, "max slope (kHz/sweep)":dbl, "funnel state":enum16{"funnel open", "funnel closed"}}
  T2 = typedef "monitor state.ctl" = cluster{"header - gamma":string[], "header - frequency":string[], "# of peaks":i32, "peaks OK":bool}
  T3 = typedef "peak monitor ctl - V2.ctl" = cluster{"delta":dbl, "gamma":dbl, "exp":dbl, "found?":bool, "found":dbl, "gamma found":dbl, "init linear":bool, "interpolate":enum16{"line", "force"}, "gamma-factor":dbl, "slope":dbl, "update freq?":bool, "update gamma?":bool, "acc factor":dbl, "linear interpolation state":T4, "ind":dbl, "gamma ratio":dbl, "gamma off limit?":bool, "freq off limit?":bool}
  T4 = typedef "interpolation state - real.ctl" = cluster{"requested size":i32, "Array":dbl[], "actual number of elements":i32}
  T5 = typedef "lorentzian.ctl" = cluster{"Amplitude":dbl, "omega(0)":dbl, "Gamma":dbl, "phase":dbl, "Q":dbl, "Norm  Ampl":dbl, "z (inf)":cdb, "4corners":T6}
  T6 = typedef "circle corners.ctl" = cluster{"z (-pi/2)":cdb, "z(inf)":cdb, "z (pi/2)":cdb, "z center":cdb, "z(0)":cdb, "radius":dbl}
  T7 = enum32{"Everything", "Everything else", "even more "}
  T8 = cluster{"omega out":dbl[], "win omega out":dbl[]}
  T9 = typedef "scale - offset gauge.ctl" = cluster{"scale offset":dbl, "scale range":dbl}
  T10 = typedef "complex region.ctl" = cluster{"max re":dbl, "min re":dbl, "max im":dbl, "min im":dbl, "delta re":dbl, "delta im":dbl, "center re":dbl, "delta  z":cdb, "center im":dbl, "center z":cdb, "d im":dbl, "d re":dbl, "d z":cdb}
  T11 = typedef "cursor winow.ctl" = cluster{"left":dbl, "right ":dbl, "center":dbl, "window":dbl, "cursors":i32[], "relative":i32, "absolute":i32, "fixed vertical offset":dbl, "vertical offset":dbl, "skew":dbl, "default window frac":dbl, "kind":enum16{"symmetric", "skewed", "fancy"}, "skew.left":dbl, "skew.right":dbl, "Plot ref":refnum<vi>, "wing order":enum16{"forw", "back"}}
  T12 = typedef "eventvkey.ctl" = enum16{"ASCII", "Enter", "Return", "Shift", "Ctrl", "Alt", "Cmd", "Opt", "Caps", "NumLock", "Clear", "Break", "Up", "Down", "Left", "Right", "Insert", "Delete", "Home", "End", "PageUp", "PageDown", "Escape", "Help", "Pause", "ScrollLock", "F1", "F2", "F3", "F4", "F5", "F6", "F7", "F8", "F9", "F10", "F11", "F12", "F13", "F14", "F15", "F16", "F17", "F18", "F19", "F20", "F21", "F22", "F23", "F24", "Play", "VolumeUp", "VolumeDown", "Mute", "Two Byte Char"}
  T13 = typedef "peak -- parameters -- complex fit.ctl" = cluster{"main VI path":path, "scale factor":dbl, "# of grid points":i32, "parameters: wavepacket":T14, "span":dbl, "interference ?":enum16{"cp z center", "pm zcenter", "fancy"}, "filter method":T15}
  T14 = typedef "wavepacket.ctl" = cluster{"R":dbl, "wave number":dbl, "delta k":dbl, "radii vector":dbl[], "radial section":cdb[], "wave vector":dbl, "wavepacket is":bool}
  T15 = typedef "filter method control.ctl" = enum16{"four", "five", "one", "two", "three", "zero", "minus one", "minus two"}
  T16 = typedef "countdown control.ctl" = enum16{"check", "start", "reset cont", "stop", "reset once"}
  T17 = typedef "plot refs -- filter related.ctl" = cluster{"Plot: complex plane - filter":refnum<vi>, "Plot: dz/domega":refnum<vi>, "Plot: fragment filter":refnum<vi>, "Plot: win omega":refnum<vi>, "Plot: phase":refnum<vi>, "Plot: phase around center":refnum<vi>, "Plot: complex plane":refnum<vi>, "Plot: fragment":refnum<vi>}
  T18 = typedef "cursor window action.ctl" = enum16{"balance", "h. offset change", "cursor moves", "change center", "change window", "init", "check", "reset", "set y to middle", "idle", "-write all Y", "-write left.X", "-write center.X", "-write right.X", "-write all X", "-change center", "-change window", "-change skew", "-read cursor 2", "-read cursor 1", "-read cursor 0", "-read all cursors", "-reset", "-read plot scale", "-set y to middle", "-Q: center.Y is visible", "-Q: window is visible", "-parse center.Y", "-right left from center", "-left move", "-right move", "-set center.Y", "-empty", "-set cursors to default", "-check", "-write center.Y", "-copy cursor 1", "-copy cursor 0", "-copy cursor 2", "move right", "move left", "shrink", "broaden", "skew up", "skew down", "-write plot scale", "zoom X", "change cen&win", "zoom to all data"}
  T19 = typedef "read scan file control.ctl" = cluster{"# columns":i32, "create bin file":bool, "do not filter":bool, "normalize phase":bool, "read freq units":enum16{"kHz", "Hz"}}
  T20 = typedef "monitor action.ctl" = enum16{"monitor", "interpolate", "global", "read", "overwrite", "write m file", "nothing", "eeee"}
  T21 = typedef "ctl -- name dispatcher -- action.ctl" = enum16{"peak frequency", "peak frequency DUMP", "peak gamma DUMP", "peak gamma", "peak frequency TEST", "peak gamma TEST", "ultrasonic power", "time in gamma", "set temperature ", "set temperature timer", "peak default gamma", "last scan file", "peak freq gamma TEST", "peak NAMES", "errors", "P_I_D", "P", "I", "D", "power vs time", "power vs time TIMER", "void", "power log", "set temperature - SINE", "itc ltc log", "peak - time in gamma"}
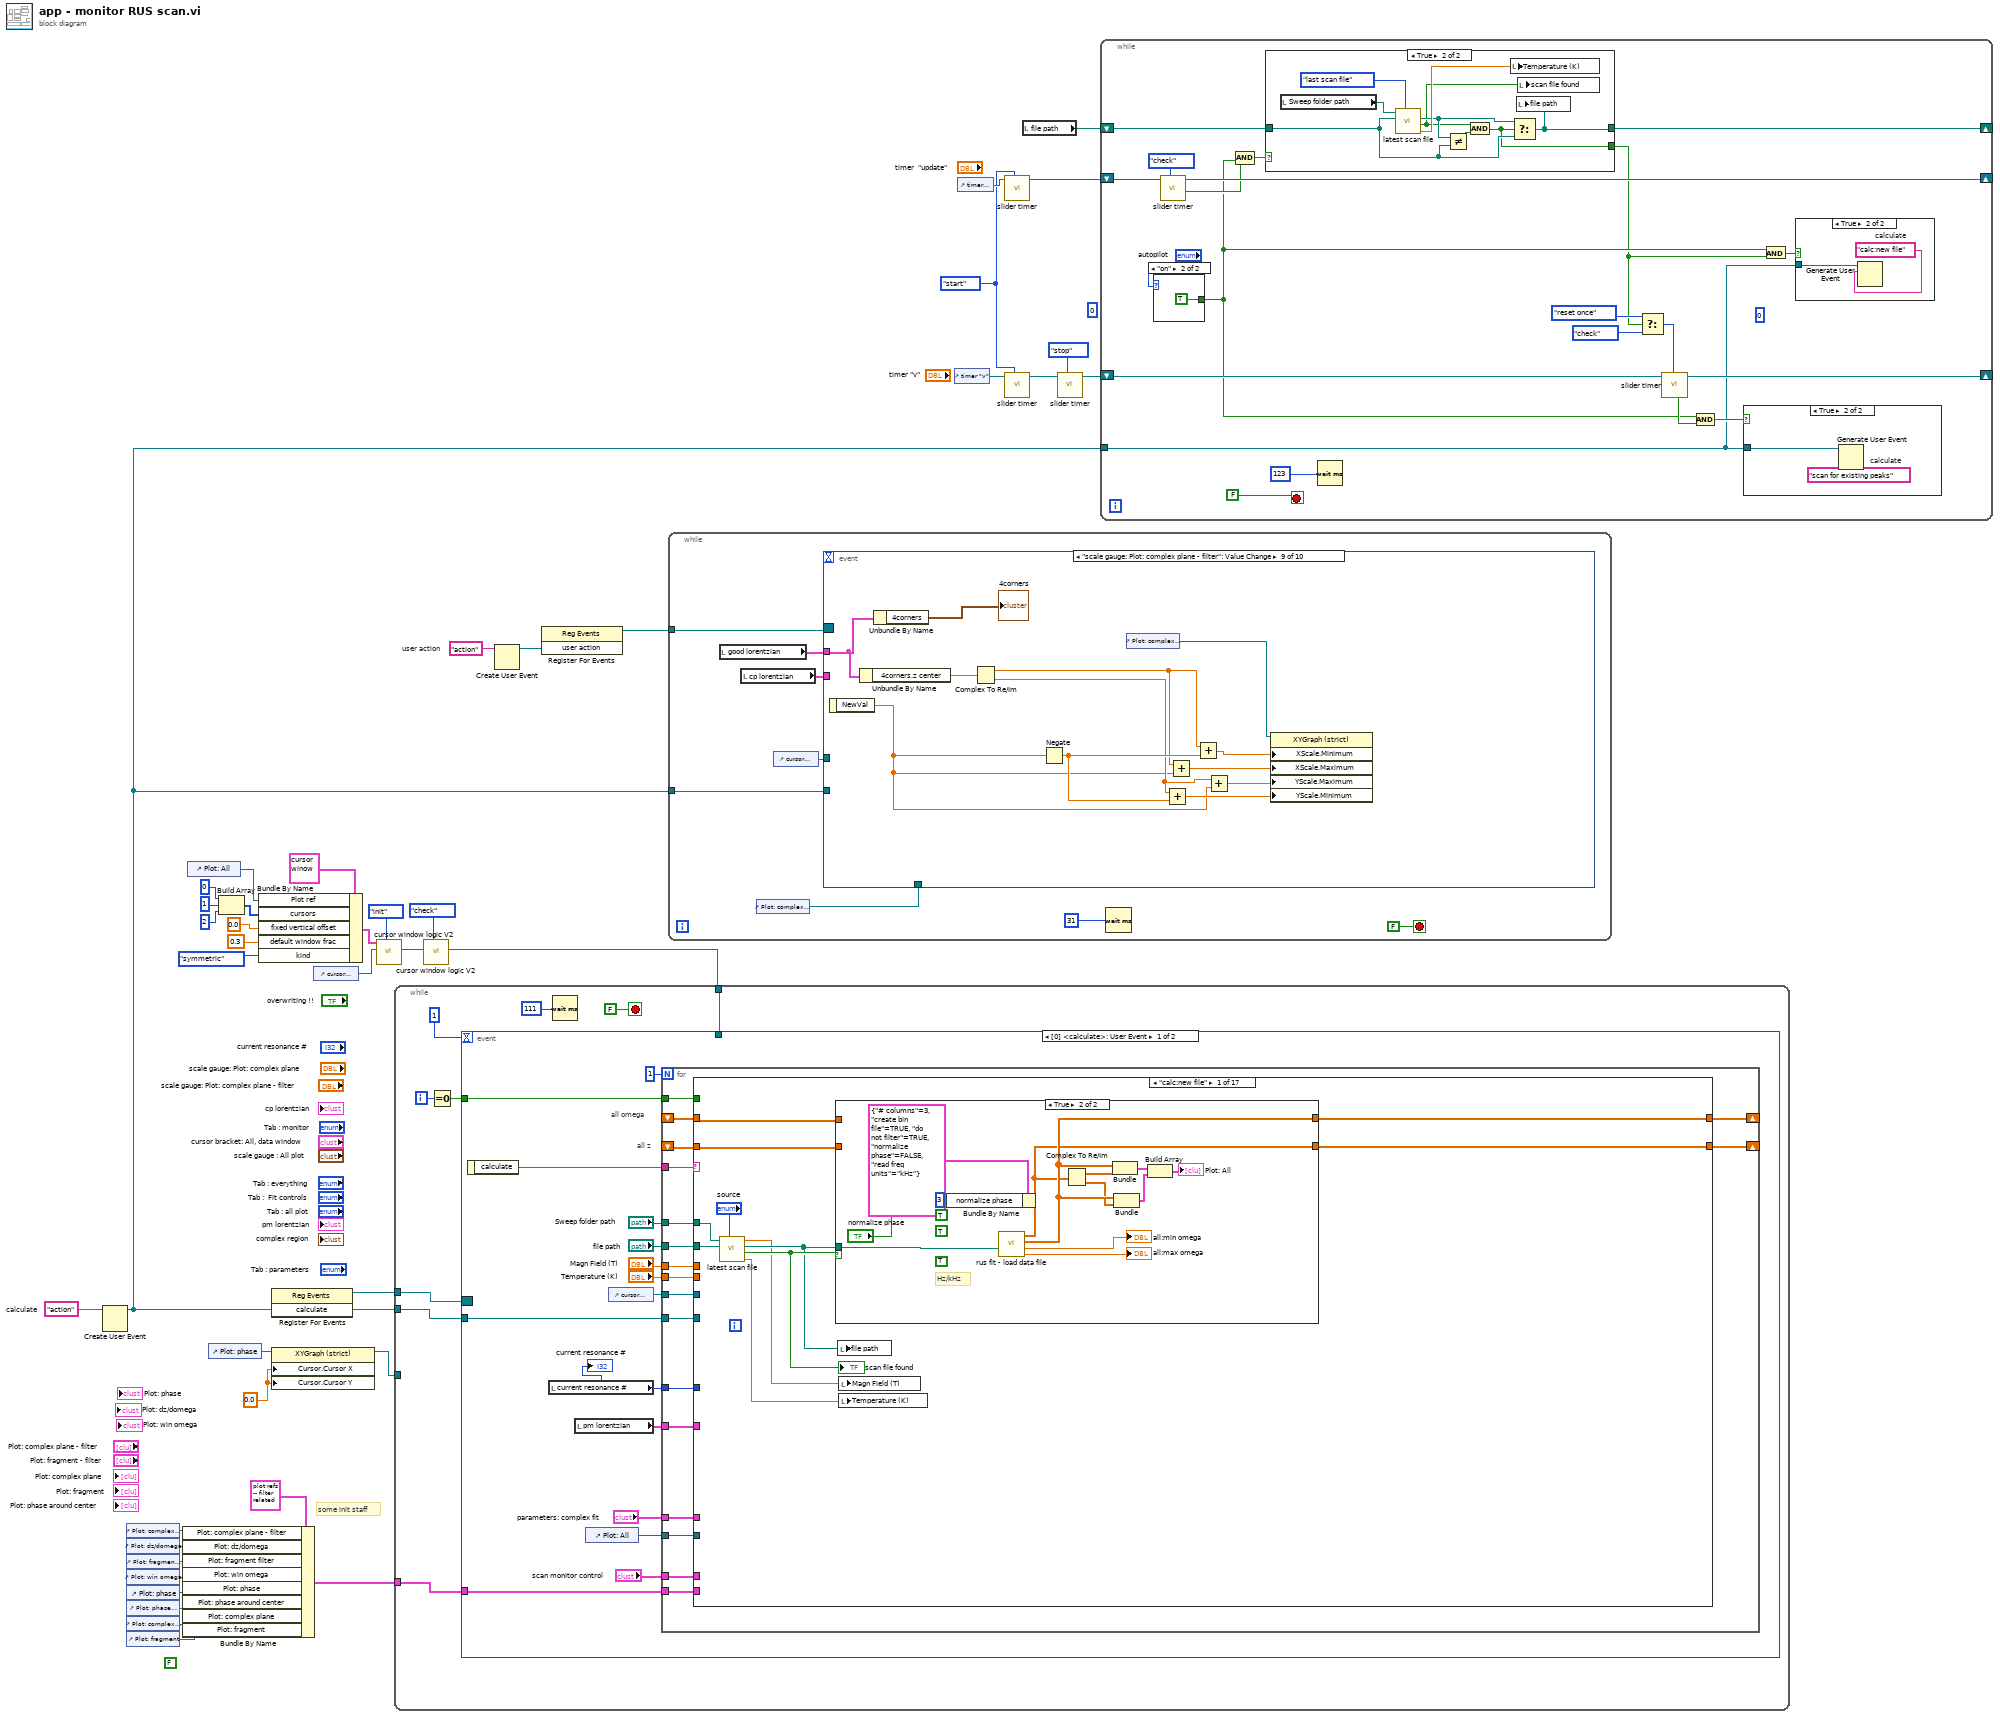
[diagram p0: block diagram]
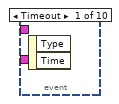
[diagram p2: hidden frame]
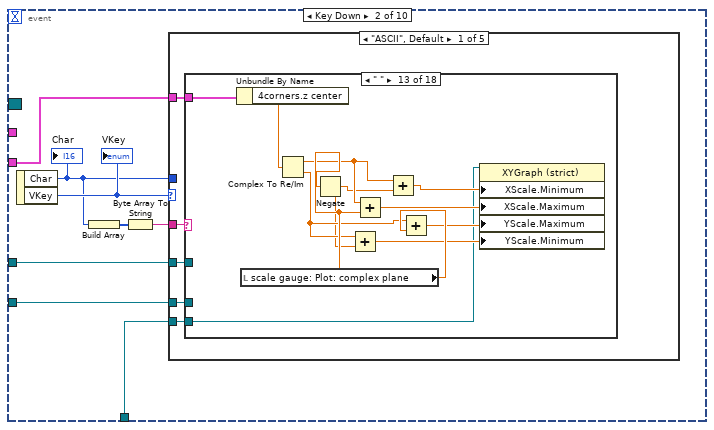
[diagram p3: hidden frame]
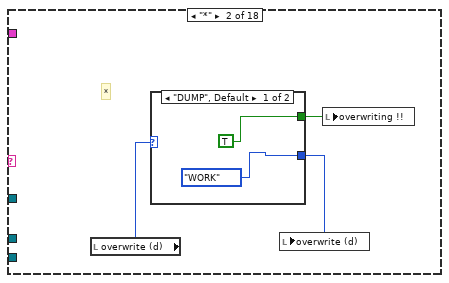
[diagram p5: hidden frame]
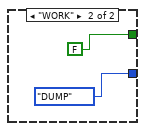
[diagram p6: hidden frame]
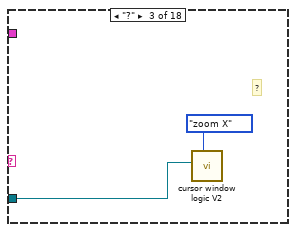
[diagram p7: hidden frame]
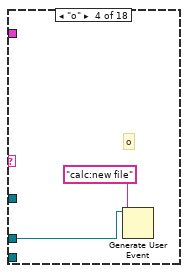
[diagram p8: hidden frame]
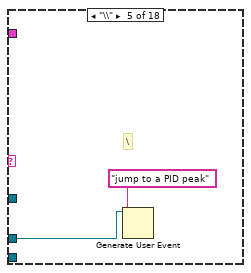
[diagram p9: hidden frame]
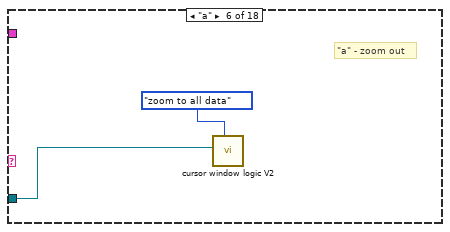
[diagram p10: hidden frame]
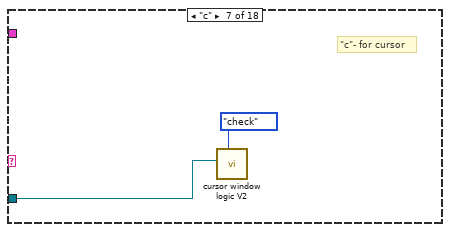
[diagram p11: hidden frame]
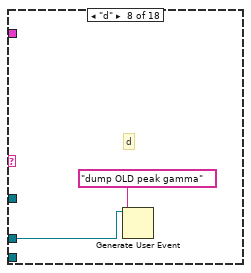
[diagram p12: hidden frame]
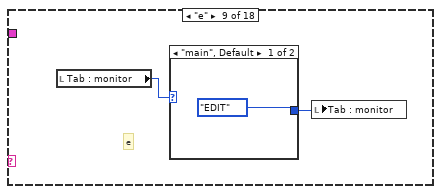
[diagram p13: hidden frame]
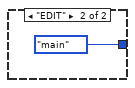
[diagram p14: hidden frame]
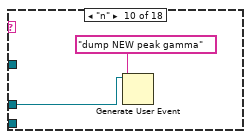
[diagram p15: hidden frame]
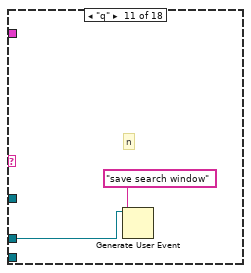
[diagram p16: hidden frame]
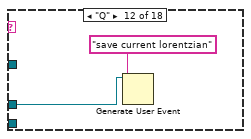
[diagram p17: hidden frame]
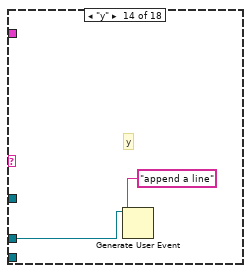
[diagram p18: hidden frame]
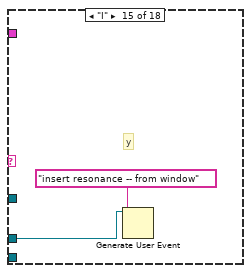
[diagram p19: hidden frame]
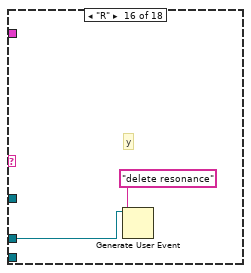
[diagram p20: hidden frame]
diagram:
  w19 = 0.0 ("Cursor.Cursor Position:Cursor X")
  w27 = "action"  # user action
  w6 = countdown_control."start" ("action")
  (unwired) 0
  w41 = "action"  # calculate
  (unwired) FALSE
  # "some init staff"
  n1 = Create User Event(user event datatype=w41) -> (user event=w25:refnum<user-event>)  [unwired: 1 in, 1 out]
  n2 = control-ref of="Plot: complex plane - filter"() -> (w16:refnum<vi>)
  n3 = control-ref of="Plot: dz/domega"() -> (w15:refnum<vi>)
  n4 = control-ref of="Plot: fragment - filter"() -> (w14:refnum<vi>)
  n5 = control-ref of="Plot: win omega"() -> (w13:refnum<vi>)
  n6 = control-ref of="Plot: phase"() -> (w12:refnum<vi>)
  n7 = control-ref of="Plot: phase around center"() -> (w10:refnum<vi>)
  n8 = control-ref of="Plot: complex plane"() -> (w9:refnum<vi>)
  n9 = control-ref of="Plot: fragment"() -> (w8:refnum<vi>)
  n10 = Bundle By Name(cluster=T17 {"Plot: complex plane - filter"=refnum, "Plot: dz/domega"=refnum, "Plot: fragment filter"=refnum, "Plot: win omega"=refnum, "Plot: phase"=refnum, "Plot: phase around center"=refnum, "Plot: complex plane"=refnum, "Plot: fragment"=refnum} ("plots: filter related"), "Plot: complex plane - filter"=w16, "Plot: dz/domega"=w15, "Plot: fragment filter"=w14, "Plot: win omega"=w13, "Plot: phase"=w12, "Plot: phase around center"=w10, "Plot: complex plane"=w9, "Plot: fragment"=w8) -> (w11:T17)
  n11 = control-ref of="Plot: All"() -> (w32:refnum<vi>)
  n12 = control-ref of="Plot: phase"() -> (w20:refnum<vi>)
  n13 = Build Array(0, 1, 2) -> (w40:i32[])
  n14 = Bundle By Name(cluster=T11 {"left"=0.0, "right "=0.0, "center"=0.0, "window"=0.0, "cursors"=[], "relative"=0, "absolute"=0, "fixed vertical offset"=0.0, "vertical offset"=0.0, "skew"=0.0, "default window frac"=0.0, "kind"=enum."symmetric", "skew.left"=0.0, "skew.right"=0.0, "Plot ref"=refnum, "wing order"=enum."forw"} ("cursor bracket: All, data window"), "Plot ref"=w32, "cursors"=w40, "fixed vertical offset"=0.0, "default window frac"=0.3 ("fixed vertical offset"), "kind"=enum16{"symmetric", "skewed", "fancy"}."symmetric") -> (w31:T11)
  n15 = register-events(w25) -> (reference out=w42:refnum<event-registration>)  [unwired: 2 in, 1 out]
  n16 = property class="XYGraph (strict)"(reference=w20, "Cursor.Cursor X"=w19, "Cursor.Cursor Y"=w19) -> (reference out=w18:refnum<vi>)  [unwired: 1 in, 1 out]
  n17 = control-ref of="cursor bracket: All, data window"() -> (w30:refnum<vi>)
  n18 = call "cursor window logic V2.vi"("cursor window action"=cursor_window_action."init", "cursor window in"=w30, "cursor window init"=w31) -> ("cursor window out"=w23:refnum<vi>)  [unwired: 7 in, 1 out]
  n19 = call "cursor window logic V2.vi"("cursor window action"=cursor_window_action."check", "cursor window in"=w23) -> ("cursor window out"=w21:refnum<vi>)  [unwired: 8 in, 1 out]
  n20 = while {
    tunnel: w42 -> [w51]
    tunnel: w25 -> [w49]
    tunnel: w21 -> [w45]
    tunnel: w18 -> [_]
    tunnel: w11 -> [w44]
    i -> [w46]
    stop <- FALSE stop-if-true
    n21 = Equal To 0?(x=w46) -> (x = 0?=w43:bool)
    n22 = event shown="[0] <calculate>: User Event" {
      selector: w51 -> [_ _]
      dyn-events: _ -> [_ _]
      timeout: 1 -> [_ _]
      tunnel: w49 -> [w65 _]
      tunnel: w45 -> [_ _]
      tunnel: w44 -> [w60 _]
      tunnel: w43 -> [w59 _]
      event User Event {
        # "all z"
        # "all omega"
        n23 = event-data() -> ("calculate"=w66:string)  [unwired: 1 in]
        n24 = local read "current resonance #"() -> (w52:i32)
        "current resonance #" <- w52
        n25 = local read "pm lorentzian"() -> (w53:T5)
        n26 = control-ref of="Plot: All"() -> (w63:refnum<vi>)
        n27 = control-ref of="cursor bracket: All, data window"() -> (w54:refnum<vi>)
        n28 = for {
          N: 1 -> [_]
          tunnel: w66 -> [w84]
          tunnel: w65 -> [w83]
          shift-right: [w80] -> _
          shift-left: _ -> [w82]
          shift-right: [w79] -> _
          shift-left: _ -> [w81]
          tunnel: w54 -> [w78]
          tunnel: w63 -> [w77]
          tunnel: "Sweep folder path" -> [w76]
          tunnel: "Temperature (K)" -> [w75]
          tunnel: w52 -> [w74]
          tunnel: w60 -> [w73]
          tunnel: w59 -> [w72]
          tunnel: "parameters: complex fit" -> [w71]
          tunnel: "file path" -> [w70]
          tunnel: "scan monitor control" -> [w69]
          tunnel: "Magn Field (T)" -> [w68]
          tunnel: w53 -> [w67]
          n29 = case shown="\"calc:new file\"" w84 {
            tunnel: w83 -> [_ _ _ _ _ _ _ _ _ _ _ w309 w327 w342 w356 _ _]
            tunnel: w82 -> [w91 w149 w197 w212 w240 w245 w257 w273 w284 w293 w295 w308 w326 w341 w355 w369 w378]
            tunnel: w81 -> [w90 w148 w196 w211 w239 w244 w256 w272 w283 w292 w294 w307 w325 w340 w354 w368 w377]
            tunnel: [w95 w149 w197 w212 w240 w245 w257 w273 w284 w293 w295 w308 w326 w341 w355 w369 w378] -> w80
            tunnel: [w94 w148 w196 w211 w239 w244 w256 w272 w283 w292 w294 w307 w325 w340 w354 w368 w377] -> w79
            tunnel: w78 -> [_ w147 _ _ w241 _ _ _ _ _ _ w310 w328 w343 w357 _ _]
            tunnel: w77 -> [_ _ _ _ _ _ _ _ _ _ _ _ _ _ _ _ _]
            tunnel: w76 -> [w93 w117 w193 w210 _ _ _ _ _ _ _ _ _ _ _ w362 w397]
            tunnel: w75 -> [_ w116 w189 w209 _ _ _ _ _ _ _ _ _ _ _ w360 _]
            tunnel: w74 -> [_ _ _ _ _ w243 w254 w266 w275 w286 _ w306 w324 w339 w345 _ _]
            tunnel: w73 -> [_ w146 _ _ w234 _ _ _ _ _ _ _ _ _ _ _ _]
            tunnel: w72 -> [_ w138 _ _ _ _ _ _ _ _ _ _ _ _ _ _ _]
            tunnel: w71 -> [_ w145 _ _ w233 _ _ _ _ _ _ _ _ _ _ _ _]
            tunnel: w70 -> [w87 _ _ _ _ _ _ _ _ _ _ _ _ _ _ _ _]
            tunnel: w69 -> [_ w114 _ _ _ _ _ _ _ _ _ _ _ _ _ _ _]
            tunnel: w68 -> [_ w113 _ _ _ _ _ _ _ _ _ _ _ _ _ _ _]
            tunnel: w67 -> [_ _ _ _ _ _ w255 w271 w282 w291 _ _ _ _ _ _ _]
            frame "calc:new file" {
              n30 = call "latest scan file.vi"("source"="source", "file path in"=w87, "sweep folder"=w93) -> ("temperature (K)"=w89:dbl, "file or folder exists?"=w92:bool, "file path out"=w88:path, "Magn Field (T)"=w85:dbl)  [unwired: 5 in]
              "scan file found" <- w92
              n31 = case shown="True" w92 {
                tunnel: [w97 w110] -> w95
                tunnel: [w96 w109] -> w94
                tunnel: w88 -> [_ w108]
                tunnel: w91 -> [w97 _]
                tunnel: w90 -> [w96 _]
                frame False {
                }
                frame True {
                  (unwired) TRUE ("read freq in")
                  (unwired) TRUE ("phase is normalized")
                  (unwired) 3 ("# columns in bin file")
                  (unwired) TRUE ("create bin file from dat")
                  # "Hz/kHz"
                  n32 = Bundle By Name(cluster=T19 {"# columns"=3, "create bin file"=TRUE, "do not filter"=TRUE, "normalize phase"=FALSE, "read freq units"=enum."kHz"} ("read scan file"), "normalize phase"="normalize phase") -> (w99:T19)
                  n33 = call "rus fit - load data file.vi"("file path"=w108, "read scan file"=w99) -> ("all:max omega"=→"all:max omega":dbl, "all:min omega"=→"all:min omega":dbl, "omega"=w110:dbl[], "x + iy"=w109:cdb[])  [unwired: 5 in, 1 out]
                  n34 = Complex To Re/Im(x + iy=w109) -> (x=w102:dbl[], y=w101:dbl[])
                  n35 = Bundle("omega"=w110, w102) -> (w103:cluster{"omega":dbl[], dbl[]})  [unwired: 1 in]
                  n36 = Bundle("omega"=w110, w101) -> (w104:cluster{"omega":dbl[], dbl[]})  [unwired: 1 in]
                  n37 = Build Array(w103, w104) -> (→"Plot: All":cluster{"omega":dbl[], dbl[]}[])
                }
              }
              n38 = local write "file path"(w88) -> ()
              n39 = local write "Magn Field (T)"(w85) -> ()
              n40 = local write "Temperature (K)"(w89) -> ()
            }
            frame "scan for existing peaks" {
              (unwired) 0 ("length")
              (unwired) 1.0 ("element")
              n41 = local read "Array of states"() -> (w144:T3[])
              n42 = local read "monitor state"() -> (w126:T2)
              n43 = Unbundle By Name(w114) -> ("iterate #"=w139:i32)
              n44 = call "monitor scan logic.vi"("Array IN"=w144, "monitor action"=monitor_action."read", "monitor state"=w126, "scan monitor control IN"=w114, "Sweep folder path"=w117, "temperature"=w116) -> ("Array OUT"=w129:T3[], "freq OUT"=w127:dbl[], "gamma OUT"=w128:dbl[], "monitor state OUT"=w134:T2)  [unwired: 6 in]
              n45 = call "monitor scan logic.vi"("Array IN"=w129, "monitor action"=monitor_action."global", "freq IN"=w127, "gamma IN"=w128, "monitor state"=w134, "scan monitor control IN"=w114) -> ("Array OUT"=w137:T3[], "freq OUT"=w136:dbl[], "gamma OUT"=w135:dbl[], "monitor state OUT"=w133:T2)  [unwired: 6 in]
              n46 = for {
                N: w139 -> [_]
                tunnel: w149 -> [w165]
                tunnel: w148 -> [w164]
                tunnel: w147 -> [w163]
                tunnel: w146 -> [w158]
                tunnel: w145 -> [w157]
                tunnel: w114 -> [w156]
                shift-right: [w154] -> w142
                shift-left: w136 -> [w161]
                shift-right: [w160] -> w141
                shift-left: w135 -> [w155]
                shift-right: [w159] -> w140
                shift-left: w137 -> [w153]
                shift-right: [w152] -> w132
                shift-left: w133 -> [w152]
                tunnel: "plot staff" -> [w151]
                tunnel: monitor_action."monitor" ("monitor action") -> [w150]
                n47 = for {
                  tunnel: w161 -> [w182] mode=indexing
                  tunnel: w163 -> [w185]
                  tunnel: w165 -> [w177]
                  tunnel: w164 -> [w176]
                  tunnel: [w183] -> w162 mode=indexing
                  tunnel: w155 -> [w179] mode=indexing
                  tunnel: w158 -> [w174]
                  tunnel: w157 -> [w173]
                  tunnel: w153 -> [w169] mode=indexing
                  tunnel: w151 -> [w167]
                  n48 = Unbundle By Name(w169) -> ("gamma-factor"=w168:dbl)
                  n49 = Multiply(x=w168, y=w179) -> (x*y=w181:dbl)
                  n50 = call "cursor window logic V2.vi"("cursor window action"=cursor_window_action."change cen&win", "window"=w181, "center"=w182, "cursor window in"=w185) -> ("cursor window out"=w170:T11)  [unwired: 6 in, 1 out]
                  n51 = call "peak -- find -- pm - V1.vi"("omega in"=w177, "z in"=w176, "cursor window"=w170, "parameters: complex fit"=w173, "plots: filter related"=w174, "plot staff ?"=w167) -> ("# points in window"=→"# of points in window":dbl, "good lorentzian"=w171:T5, "pm lorentzian"=w178:T5, "cp lorentzian"=w172:T5)  [unwired: 10 in]
                  n52 = Unbundle By Name(w171) -> ("omega(0)"=w175:dbl, "Gamma"=w180:dbl)
                  n53 = local write "pm lorentzian"(w178) -> ()
                  n54 = local write "cp lorentzian"(w172) -> ()
                  n55 = Bundle By Name(cluster=w169, "exp"=w182, "found"=w175, "gamma"=w179, "gamma found"=w180) -> (w183:T3)
                }
                n56 = call "monitor scan logic.vi"("Array IN"=w162, "monitor action"=w150, "scan monitor control IN"=w156) -> ("Array OUT"=w159:T3[], "freq OUT"=w154:dbl[], "gamma OUT"=w160:dbl[])  [unwired: 9 in, 1 out]
              }
              n57 = local write "OLD gamma"(w128) -> ()
              n58 = local write "OLD freq"(w127) -> ()
              n59 = call "monitor scan logic.vi"("Array IN"=w140, "monitor action"=monitor_action."interpolate", "init"=w138, "freq IN"=w142, "gamma IN"=w141, "monitor state"=w132, "scan monitor control IN"=w114) -> ("Array OUT"=w125:T3[], "freq OUT"=w123:dbl[], "gamma OUT"=w122:dbl[], "monitor state OUT"=w121:T2)  [unwired: 5 in]
              n60 = call "monitor scan logic.vi"("Array IN"=w125, "monitor action"=monitor_action."overwrite", "freq IN"=w123, "Magn Field (T)"=w113, "gamma IN"=w122, "monitor state"=w121, "scan monitor control IN"=w114, "Sweep folder path"=w117, "temperature"=w116) -> ("Array OUT"=w124:T3[], "freq OUT"=w118:dbl[], "gamma OUT"=w119:dbl[], "monitor state OUT"=w120:T2)  [unwired: 3 in]
              n61 = local write "Array of states"(w124) -> ()
              n62 = local write "NEW freq"(w118) -> ()
              n63 = local write "NEW gamma"(w119) -> ()
              n64 = local write "monitor state"(w120) -> ()
            }
            frame "dump OLD peak gamma" {
              w192 = enum16{"append", "overwrite"}."overwrite" ("append/overwrite")
              n65 = local read "OLD gamma"() -> (w190:dbl[])
              n66 = local read "OLD freq"() -> (w194:dbl[])
              n67 = case shown="\"WORK\"" "overwrite (d)" {
                tunnel: [ctl_--_name_dispatcher_--_action."peak frequency DUMP" ("ctl name dispatch") ctl_--_name_dispatcher_--_action."peak frequency" ("ctl name dispatch")] -> w195
                tunnel: [ctl_--_name_dispatcher_--_action."peak gamma DUMP" ("ctl name dispatch") ctl_--_name_dispatcher_--_action."peak gamma" ("ctl name dispatch")] -> w191
                tunnel: [enum16{"DUMP", "WORK", ""}."DUMP" ("dump/work") enum16{"DUMP", "WORK", ""}."DUMP" ("dump/work")] -> w187
                tunnel: [FALSE ("overwriting !!") FALSE ("overwriting !!")] -> w186
                frame "DUMP", Default {
                }
                frame "WORK" {
                }
              }
              n68 = call "PID append overwrite.vi"("temperature"=w189, "append/overwrite"=w192, "PID freq"=w194, "ctl kind IN"=w195, "sweep folder"=w193) -> ()  [unwired: 6 in, 1 out]
              n69 = call "PID append overwrite.vi"("temperature"=w189, "append/overwrite"=w192, "PID freq"=w190, "ctl kind IN"=w191, "sweep folder"=w193) -> ()  [unwired: 6 in, 1 out]
              n70 = local write "overwriting !!"(w186) -> ()
              n71 = local write "overwrite (d)"(w187) -> ()
            }
            frame "dump NEW peak gamma" {
              n72 = case shown="True" TRUE {
                tunnel: w210 -> [_ w221]
                tunnel: w209 -> [_ w220]
                frame False {
                }
                frame True {
                  w217 = enum16{"append", "overwrite"}."overwrite" ("append/overwrite")
                  n73 = local read "NEW gamma"() -> (w215:dbl[])
                  n74 = local read "NEW freq"() -> (w218:dbl[])
                  n75 = case shown="\"DUMP\", Default" "dump/work NEW (\"n\")" {
                    tunnel: [ctl_--_name_dispatcher_--_action."peak frequency DUMP" ("ctl name dispatch") ctl_--_name_dispatcher_--_action."peak frequency" ("ctl name dispatch")] -> w219
                    tunnel: [ctl_--_name_dispatcher_--_action."peak gamma DUMP" ("ctl name dispatch") ctl_--_name_dispatcher_--_action."peak gamma" ("ctl name dispatch")] -> w216
                    tunnel: [enum16{"DUMP", "WORK", ""}."DUMP" ("dump/work") enum16{"DUMP", "WORK", ""}."DUMP" ("dump/work")] -> w213
                    frame "DUMP", Default {
                    }
                    frame "WORK" {
                    }
                  }
                  n76 = call "PID append overwrite.vi"("temperature"=w220, "append/overwrite"=w217, "PID freq"=w218, "ctl kind IN"=w219, "sweep folder"=w221) -> ()  [unwired: 6 in, 1 out]
                  n77 = local write "dump/work NEW (\"n\")"(w213) -> ()
                  n78 = call "PID append overwrite.vi"("temperature"=w220, "append/overwrite"=w217, "PID freq"=w215, "ctl kind IN"=w216, "sweep folder"=w221) -> ()  [unwired: 6 in, 1 out]
                }
              }
              n79 = local read "NEW gamma"() -> (w208:dbl[])
              n80 = local read "NEW freq"() -> (w207:dbl[])
              n81 = local write "OLD gamma"(w208) -> ()
              n82 = local write "OLD freq"(w207) -> ()
            }
            frame "one peak" {
              n83 = call "cursor window logic V2.vi"("cursor window action"=cursor_window_action."check", "cursor window in"=w241) -> ("cursor window out"=w238:T11)  [unwired: 8 in, 1 out]
              n84 = Unbundle By Name(w238) -> ("center"=→"window center (kHz)":dbl, "window"=→"window width (kHz)":dbl)
              n85 = call "peak -- find -- pm - V1.vi"("omega in"=w240, "z in"=w239, "cursor window"=w238, "parameters: complex fit"=w233, "plots: filter related"=w234, "plot staff ?"=enum16{"plot", "do not plot", "a"}."plot", "just guess?"="use fast fit?") -> ("# points in window"=w231:dbl, "good lorentzian"=→"good lorentzian":T5, "pm lorentzian"=w235:T5, "cp lorentzian"=w232:T5)  [unwired: 9 in]
              n86 = local write "# of points in window"(w231) -> ()
              n87 = local write "pm lorentzian"(w235) -> ()
              n88 = local write "cp lorentzian"(w232) -> ()
            }
            frame "save search window" {
              n89 = local read "OLD gamma"() -> (w248:dbl[])
              n90 = local read "OLD freq"() -> (w249:dbl[])
              n91 = in-place {
                n92 = in-place-array #1(w249, w243) -> ()  [unwired: 1 out]
                n93 = local read "window center (kHz)"() -> (w251:dbl)
                n94 = in-place-array #1(w251) -> (w246:dbl[])  [unwired: 1 out]
              }
              n95 = in-place {
                n96 = in-place-array #2(w248, w243) -> ()  [unwired: 1 out]
                n97 = local read "window width (kHz)"() -> (w250:dbl)
                n98 = in-place-array #2(w250) -> (w247:dbl[])  [unwired: 1 out]
              }
              n99 = local write "OLD freq"(w246) -> ()
              n100 = local write "OLD gamma"(w247) -> ()
            }
            frame "save current lorentzian" {
              n101 = local read "OLD gamma"() -> (w260:dbl[])
              n102 = local read "OLD freq"() -> (w261:dbl[])
              n103 = Unbundle By Name(w255) -> ("omega(0)"=w253:dbl, "Gamma"=w252:dbl)
              n104 = in-place {
                in-place-border: w253 -> [w263]
                n105 = in-place-array #3(w261, w254) -> ()  [unwired: 1 out]
                n106 = in-place-array #3(w263) -> (w258:dbl[])  [unwired: 1 out]
              }
              n107 = in-place {
                in-place-border: w252 -> [w262]
                n108 = in-place-array #4(w260, w254) -> ()  [unwired: 1 out]
                n109 = in-place-array #4(w262) -> (w259:dbl[])  [unwired: 1 out]
              }
              n110 = local write "OLD freq"(w258) -> ()
              n111 = local write "OLD gamma"(w259) -> ()
            }
            frame "insert resonance -- from lorentzian" {
              n112 = local read "OLD gamma"() -> (w268:dbl[])
              n113 = local read "OLD freq"() -> (w270:dbl[])
              n114 = Unbundle By Name(w271) -> ("omega(0)"=w265:dbl, "Gamma"=w264:dbl)
              n115 = Insert Into Array(array=w270, index=w266, new element=w265) -> (w269:dbl[])
              n116 = Insert Into Array(array=w268, index=w266, new element=w264) -> (w267:dbl[])
              n117 = local write "OLD freq"(w269) -> ()
              n118 = local write "OLD gamma"(w267) -> ()
            }
            frame "insert resonance -- from window" {
              n119 = local read "window center (kHz)"() -> (w280:dbl)
              n120 = local read "window width (kHz)"() -> (w276:dbl)
              n121 = local read "OLD gamma"() -> (w278:dbl[])
              n122 = local read "OLD freq"() -> (w281:dbl[])
              n123 = Unbundle By Name(w282) -> ()  [unwired: 2 out]
              n124 = call "array -- incert after.vi"("index"=w275, "Array"=w281, "number"=w280) -> ("array out"=w279:dbl[])  [unwired: 7 in, 1 out]
              n125 = call "array -- incert after.vi"("index"=w275, "Array"=w278, "number"=w276) -> ("array out"=w277:dbl[], "new index"=w274:i32)  [unwired: 7 in]
              n126 = local write "OLD freq"(w279) -> ()
              n127 = local write "OLD gamma"(w277) -> ()
              n128 = local write "current resonance #"(w274) -> ()
            }
            frame "delete resonance" {
              w285 = 1 ("length")
              n129 = local read "OLD gamma"() -> (w288:dbl[])
              n130 = local read "OLD freq"() -> (w290:dbl[])
              n131 = Unbundle By Name(w291) -> ()  [unwired: 2 out]
              n132 = Delete From Array(array=w290, length=w285, index=w286) -> (array with subset deleted=w289:dbl[])  [unwired: 1 out]
              n133 = Delete From Array(array=w288, length=w285, index=w286) -> (array with subset deleted=w287:dbl[])  [unwired: 1 out]
              n134 = local write "OLD freq"(w289) -> ()
              n135 = local write "OLD gamma"(w287) -> ()
            }
            frame "aaa", Default {
            }
            frame "jump to a PID peak" {
              w297 = "one peak"  # event data
              n136 = local read "OLD freq"() -> (w311:dbl[])
              n137 = case shown="True" TRUE {
                tunnel: w306 -> [w312 w314]
                tunnel: [w312 w313] -> w305
                frame False {
                }
                frame True {
                  n138 = Increment(x=w314) -> (x+1=w313:i32)
                }
              }
              n139 = Generate User Event(user event=w309, event data cluster=w297) -> ()  [unwired: 2 in, 2 out]
              n140 = Array Size(array=w311) -> (size(s)=w302:i32)
              n141 = Equal To 0?(x=w302) -> (x = 0?=w304:bool)
              n142 = Select(t=1, s=w304, f=w302) -> (s? t:f=w301:i32)
              n143 = Quotient & Remainder(x=w305, y=w301) -> (x-y*floor(x/y)=w298:i32)  [unwired: 1 out]
              n144 = local write "current resonance #"(w298) -> ()
              n145 = Index Array(array=w311, index=w298) -> (element=w299:dbl)
              n146 = call "cursor window logic V2.vi"("cursor window action"=cursor_window_action."change center", "center"=w299, "cursor window in"=w310) -> ()  [unwired: 7 in, 2 out]
            }
            frame "next resonance" {
              (unwired) TRUE
              w315 = "one peak"  # event data
              n147 = local read "OLD freq"() -> (w329:dbl[])
              n148 = Generate User Event(user event=w327, event data cluster=w315) -> ()  [unwired: 2 in, 2 out]
              n149 = Increment(x=w324) -> (x+1=w323:i32)
              n150 = Array Size(array=w329) -> (size(s)=w320:i32)
              n151 = Equal To 0?(x=w320) -> (x = 0?=w322:bool)
              n152 = Select(t=1, s=w322, f=w320) -> (s? t:f=w319:i32)
              n153 = Quotient & Remainder(x=w323, y=w319) -> (x-y*floor(x/y)=w316:i32)  [unwired: 1 out]
              n154 = local write "current resonance #"(w316) -> ()
              n155 = Index Array(array=w329, index=w316) -> (element=w317:dbl)
              n156 = call "cursor window logic V2.vi"("cursor window action"=cursor_window_action."change center", "center"=w317, "cursor window in"=w328) -> ()  [unwired: 7 in, 2 out]
            }
            frame "prev resonance" {
              (unwired) TRUE
              w330 = "one peak"  # event data
              n157 = local read "OLD freq"() -> (w344:dbl[])
              n158 = Generate User Event(user event=w342, event data cluster=w330) -> ()  [unwired: 2 in, 2 out]
              n159 = Decrement(x=w339) -> (x-1=w338:i32)
              n160 = Array Size(array=w344) -> (size(s)=w335:i32)
              n161 = Equal To 0?(x=w335) -> (x = 0?=w337:bool)
              n162 = Select(t=1, s=w337, f=w335) -> (s? t:f=w334:i32)
              n163 = Quotient & Remainder(x=w338, y=w334) -> (x-y*floor(x/y)=w331:i32)  [unwired: 1 out]
              n164 = local write "current resonance #"(w331) -> ()
              n165 = Index Array(array=w344, index=w331) -> (element=w332:dbl)
              n166 = call "cursor window logic V2.vi"("cursor window action"=cursor_window_action."change center", "center"=w332, "cursor window in"=w343) -> ()  [unwired: 7 in, 2 out]
            }
            frame "jump to a resonance" {
              (unwired) TRUE
              w346 = "one peak"  # event data
              n167 = local read "OLD freq"() -> (w358:dbl[])
              n168 = Generate User Event(user event=w356, event data cluster=w346) -> ()  [unwired: 2 in, 2 out]
              n169 = Array Size(array=w358) -> (size(s)=w351:i32)
              n170 = Equal To 0?(x=w351) -> (x = 0?=w353:bool)
              n171 = Select(t=1, s=w353, f=w351) -> (s? t:f=w350:i32)
              n172 = Quotient & Remainder(x=w345, y=w350) -> (x-y*floor(x/y)=w347:i32)  [unwired: 1 out]
              n173 = local write "current resonance #"(w347) -> ()
              n174 = Index Array(array=w358, index=w347) -> (element=w348:dbl)
              n175 = call "cursor window logic V2.vi"("cursor window action"=cursor_window_action."change center", "center"=w348, "cursor window in"=w357) -> ()  [unwired: 7 in, 2 out]
            }
            frame "reread resonances" {
              (unwired) TRUE
              n176 = call "PID -- read interpolate.vi"("sweep folder path"=w362, "ctl PID file IN"=ctl_--_name_dispatcher_--_action."peak frequency" ("ctl name dispatch"), "temperature"=w360) -> ("sweep folder path out"=w366:path, "PID freq"=w361:dbl[], "length out"=w363:i32)  [unwired: 11 in, 3 out]
              n177 = call "PID -- read interpolate.vi"("sweep folder path"=w366, "ctl PID file IN"=ctl_--_name_dispatcher_--_action."peak gamma" ("ctl name dispatch"), "length"=w363, "default"=1.0 ("element")) -> ("PID freq"=w359:dbl[])  [unwired: 10 in, 5 out]
              n178 = local write "OLD gamma"(w359) -> ()
              n179 = local write "OLD freq"(w361) -> ()
            }
            frame "append a line" {
              (unwired) "ctl_PID_peak_gamma_NEW.dat" ("freq PID file IN")
              w399 = 0.0 ("lower")
              n180 = call "ctl -- name dispatcher.vi"("ctl name dispatch"=ctl_--_name_dispatcher_--_action."peak frequency TEST") -> ("ctl file name"=w374:string)  [unwired: 8 in, 2 out]
              n181 = call "ctl -- name dispatcher.vi"("ctl name dispatch"=ctl_--_name_dispatcher_--_action."peak gamma TEST") -> ("ctl file name"=w372:string)  [unwired: 8 in, 2 out]
              n182 = local read "pm lorentzian"() -> (w402:T5)
              n183 = call "ctl -- name dispatcher.vi"("ctl name dispatch"=ctl_--_name_dispatcher_--_action."peak freq gamma TEST") -> ("ctl file name"=w370:string)  [unwired: 8 in, 2 out]
              n184 = call "file -- 9w path.vi"("sweep folder"=w397) -> ("9w path"=w386:path)  [unwired: 10 in]
              n185 = Unbundle By Name(w402) -> ("omega(0)"=w401:dbl, "Gamma"=w400:dbl)
              n186 = Build Path(base path=w386, name or relative path=w370) -> (appended path=w376:path)
              n187 = Build Path(base path=w386, name or relative path=w372) -> (appended path=w388:path)
              n188 = Build Path(base path=w386, name or relative path=w374) -> (appended path=w396:path)
              n189 = call "Q -- check range -- i -- real.vi"("lower"=w399, "default"=1.0, "number"=w400) -> ("number in range"=w387:dbl)  [unwired: 6 in, 2 out]
              n190 = call "Q -- check range -- i -- real.vi"("lower"=w399, "default"=w399, "number"=w401) -> ("number in range"=w394:dbl)  [unwired: 6 in, 2 out]
              n191 = Number To Fractional String(number=w387) -> (F-format string=w381:string)  [unwired: 3 in]
              n192 = Number To Fractional String(number=w394) -> (F-format string=w382:string)  [unwired: 3 in]
              n193 = Build Array(w381) -> (w390:string[])
              n194 = Build Array(w382) -> (w393:string[])
              n195 = call-poly <vilib>:"Write To Spreadsheet File.vi"("delimiter (\\t)"="\r", "append to file? (new file:F)"=TRUE, "1D data"=w390, "file path (dialog if empty)"=w388) -> ()  [unwired: 4 in, 1 out]
              n196 = call-poly <vilib>:"Write To Spreadsheet File.vi"("delimiter (\\t)"="\r", "append to file? (new file:F)"=TRUE, "1D data"=w393, "file path (dialog if empty)"=w396) -> ()  [unwired: 4 in, 1 out]
              n197 = Concatenate Strings(w382, "\t", w381) -> (w380:string)
              n198 = Build Array(w380) -> (w384:string[])
              n199 = call-poly <vilib>:"Write To Spreadsheet File.vi"("delimiter (\\t)"="\r", "append to file? (new file:F)"=TRUE, "1D data"=w384, "file path (dialog if empty)"=w376) -> ()  [unwired: 4 in, 1 out]
            }
          }
        }
      }
      event Timeout {
        n200 = event-data() -> ()  [unwired: 1 in, 2 out]
      }
    }
    n201 = Wait (ms)(milliseconds to wait=u32 111) -> ()  [unwired: 1 out]
  }
  n202 = Create User Event(user event datatype=w27) -> (user event=w26:refnum<user-event>)  [unwired: 1 in, 1 out]
  n203 = register-events(w26) -> (reference out=w28:refnum<event-registration>)  [unwired: 2 in, 1 out]
  n204 = while {
    tunnel: w28 -> [w410]
    tunnel: w25 -> [w409]
    stop <- FALSE stop-if-true
    n205 = local read "good lorentzian"() -> (w403:T5)
    n206 = local read "cp lorentzian"() -> (w406:T5)
    n207 = control-ref of="Plot: complex plane"() -> (w405:refnum<vi>)
    n208 = control-ref of="cursor bracket: All, data window"() -> (w404:refnum<vi>)
    n209 = event shown="[8] \"scale gauge: Plot: complex plane - filter\": Value Change" {
      selector: w410 -> [_ _ _ _ _ _ _ _ _ _]
      dyn-events: _ -> [_ _ _ _ _ _ _ _ _ _]
      timeout: _ -> [_ _ _ _ _ _ _ _ _ _]
      tunnel: w409 -> [_ w417 _ _ _ _ _ w534 _ _]
      tunnel: w404 -> [_ w416 _ _ _ _ w532 _ _ _]
      tunnel: w406 -> [_ w412 _ _ _ _ _ _ _ w552]
      tunnel: w405 -> [_ w411 _ _ _ _ _ _ _ w550]
      tunnel: w403 -> [_ _ _ _ _ _ _ _ w539 _]
      event Timeout {
        n210 = event-data() -> ()  [unwired: 1 in, 2 out]
      }
      event Key Down {
        n211 = event-data() -> ("Char"=w414:i16, "VKey"=w418:T12)  [unwired: 1 in]
        "Char" <- w414
        "VKey" <- w418
        n212 = Build Array(w414) -> (w415:i16[])
        n213 = Byte Array To String(unsigned byte array=w415) -> (string=w413:string)
        n214 = case shown="\"ASCII\", Default" w418 {
          selector: w418 -> [_ _ _ _ w485]
          tunnel: w414 -> [_ _ _ _ _]
          tunnel: w417 -> [w423 _ w479 w481 w484]
          tunnel: w416 -> [w422 _ _ _ w486]
          tunnel: w413 -> [w421 _ _ _ _]
          tunnel: w412 -> [w420 _ _ _ _]
          tunnel: w411 -> [w419 _ _ _ _]
          frame "ASCII", Default {
            n215 = case shown="\" \"" w421 {
              tunnel: w423 -> [_ _ _ w434 w436 _ _ w442 _ w448 w450 w452 _ w465 w467 w469 w473 w476]
              tunnel: w422 -> [_ _ w431 _ _ w437 w439 _ _ _ _ _ _ _ _ _ _ _]
              tunnel: w420 -> [_ _ _ _ _ _ _ _ _ _ _ _ w453 _ _ _ _ _]
              tunnel: w419 -> [_ _ _ _ _ _ _ _ _ _ _ _ w454 _ _ _ _ _]
              frame "0", Default {
              }
              frame "*" {
                # "*"
                n216 = local read "overwrite (d)"() -> (w426:enum16{"DUMP", "WORK", ""})
                n217 = case shown="\"DUMP\", Default" w426 {
                  tunnel: [enum16{"DUMP", "WORK", ""}."WORK" ("overwrite dump/work (\"d\")") enum16{"DUMP", "WORK", ""}."DUMP" ("overwrite dump/work (\"d\")")] -> w425
                  tunnel: [TRUE ("overwriting !!") FALSE ("overwriting !!")] -> w424
                  frame "DUMP", Default {
                  }
                  frame "WORK" {
                  }
                }
                n218 = local write "overwrite (d)"(w425) -> ()
                n219 = local write "overwriting !!"(w424) -> ()
              }
              frame "?" {
                # "?"
                n220 = call "cursor window logic V2.vi"("cursor window action"=cursor_window_action."zoom X", "cursor window in"=w431) -> ()  [unwired: 8 in, 2 out]
              }
              frame "o" {
                # "o"
                n221 = Generate User Event(user event=w434, event data cluster="calc:new file" ("event data")) -> ()  [unwired: 2 in, 2 out]
              }
              frame "\\" {
                # "\\"
                n222 = Generate User Event(user event=w436, event data cluster="jump to a PID peak" ("event data")) -> ()  [unwired: 2 in, 2 out]
              }
              frame "a" {
                # "\"a\" - zoom out"
                n223 = call "cursor window logic V2.vi"("cursor window action"=cursor_window_action."zoom to all data", "cursor window in"=w437) -> ()  [unwired: 8 in, 2 out]
              }
              frame "c" {
                # "\"c\"- for cursor"
                n224 = call "cursor window logic V2.vi"("cursor window action"=cursor_window_action."check", "cursor window in"=w439) -> ()  [unwired: 8 in, 2 out]
              }
              frame "d" {
                # "d"
                n225 = Generate User Event(user event=w442, event data cluster="dump OLD peak gamma" ("event data")) -> ()  [unwired: 2 in, 2 out]
              }
              frame "e" {
                # "e"
                n226 = local read "Tab : monitor"() -> (w444:enum32{"main", "EDIT"})
                n227 = case shown="\"main\", Default" w444 {
                  tunnel: [enum32{"main", "EDIT"}."EDIT" ("Tab : monitor") enum32{"main", "EDIT"}."main" ("Tab : monitor")] -> w443
                  frame "main", Default {
                  }
                  frame "EDIT" {
                  }
                }
                n228 = local write "Tab : monitor"(w443) -> ()
              }
              frame "n" {
                n229 = Generate User Event(user event=w448, event data cluster="dump NEW peak gamma" ("event data")) -> ()  [unwired: 2 in, 2 out]
              }
              frame "q" {
                # "n"
                n230 = Generate User Event(user event=w450, event data cluster="save search window" ("event data")) -> ()  [unwired: 2 in, 2 out]
              }
              frame "Q" {
                n231 = Generate User Event(user event=w452, event data cluster="save current lorentzian" ("event data")) -> ()  [unwired: 2 in, 2 out]
              }
              frame " " {
                n232 = Unbundle By Name(w453) -> ("4corners.z center"=w462:cdb)
                n233 = local read "scale gauge: Plot: complex plane"() -> (w463:dbl)
                n234 = Complex To Re/Im(x + iy=w462) -> (x=w461:dbl, y=w460:dbl)
                n235 = Negate(x=w463) -> (-x=w455:dbl)
                n236 = Add(x=w460, y=w455) -> (x+y=w459:dbl)
                n237 = Add(x=w461, y=w463) -> (x+y=w457:dbl)
                n238 = Add(x=w461, y=w455) -> (x+y=w456:dbl)
                n239 = Add(x=w460, y=w463) -> (x+y=w458:dbl)
                n240 = property on="Property Node" class="XYGraph (strict)"(reference=w454, "XScale.Minimum"=w456, "XScale.Maximum"=w457, "YScale.Maximum"=w458, "YScale.Minimum"=w459) -> ()  [unwired: 1 in, 2 out]
              }
              frame "y" {
                # "y"
                n241 = Generate User Event(user event=w465, event data cluster="append a line" ("event data")) -> ()  [unwired: 2 in, 2 out]
              }
              frame "I" {
                # "y"
                n242 = Generate User Event(user event=w467, event data cluster="insert resonance -- from window" ("event data")) -> ()  [unwired: 2 in, 2 out]
              }
              frame "R" {
                # "y"
                n243 = Generate User Event(user event=w469, event data cluster="delete resonance" ("event data")) -> ()  [unwired: 2 in, 2 out]
              }
              frame "U" {
                n244 = for {
                  N: 100 -> [_]
                  tunnel: [w474] -> w470 mode=indexing
                  i -> [w474]
                }
                "index" <- w470
                n245 = Generate User Event(user event=w473, event data cluster="reread resonances" ("event data")) -> ()  [unwired: 2 in, 2 out]
              }
              frame "v" {
                # "v"
                n246 = Generate User Event(user event=w476, event data cluster="scan for existing peaks" ("event data")) -> ()  [unwired: 2 in, 2 out]
              }
            }
          }
          frame "Escape" {
            n247 = local read "use fast fit?"() -> (w477:bool)
            n248 = Not(x=w477) -> (.not. x?=w478:bool)
            n249 = local write "use fast fit?"(w478) -> ()
          }
          frame "PageUp" {
            n250 = Generate User Event(user event=w479, event data cluster="next resonance" ("event data")) -> ()  [unwired: 2 in, 2 out]
          }
          frame "PageDown" {
            n251 = Generate User Event(user event=w481, event data cluster="prev resonance" ("event data")) -> ()  [unwired: 2 in, 2 out]
          }
          frame "Up".."Right" {
            n252 = case shown="\"Left\"" w485 {
              tunnel: w486 -> [w487 w489 w491 w494]
              frame "Right", Default {
                n253 = call "cursor window logic V2.vi"("cursor window action"=cursor_window_action."move right", "cursor window in"=w487) -> ()  [unwired: 8 in, 2 out]
              }
              frame "Left" {
                n254 = call "cursor window logic V2.vi"("cursor window action"=cursor_window_action."move left", "cursor window in"=w489) -> ()  [unwired: 8 in, 2 out]
              }
              frame "Up" {
                n255 = call "cursor window logic V2.vi"("cursor window action"=cursor_window_action."broaden", "cursor window in"=w491) -> ()  [unwired: 8 in, 2 out]
              }
              frame "Down" {
                n256 = call "cursor window logic V2.vi"("cursor window action"=cursor_window_action."shrink", "cursor window in"=w494) -> ()  [unwired: 8 in, 2 out]
              }
            }
            n257 = Generate User Event(user event=w484, event data cluster="one peak" ("event data")) -> ()  [unwired: 2 in, 2 out]
          }
        }
      }
      event Value Change {
        n258 = event-data() -> ("CtlRef"=w498:refnum<vi>)  [unwired: 1 in, 5 out]
        n259 = local read "scan monitor control"() -> (w496:T1)
        n260 = property class="Ctl"(reference=w498) -> ("Label.Text"=w497:string)  [unwired: 1 in, 2 out]
        n261 = case shown="\"Unique strike pars\", Default" w497 {
          tunnel: w496 -> [w500 w511]
          tunnel: [w499 w510] -> w495
          frame "Unique strike pars", Default {
            n262 = in-place {
              n263 = in-place-cluster #5(w500) -> ("Unique strike parameters"=w504:bool)  [unwired: 1 out]
              n264 = Not(x=w504) -> (.not. x?=w503:bool)
              n265 = case shown="True" w503 {
                selector: w503 -> [w507 w508]
                tunnel: [enum16{"funnel open", "funnel closed"}."funnel open" ("funnel state") enum16{"funnel open", "funnel closed"}."funnel closed" ("funnel state")] -> w505
                tunnel: [w507 w508] -> w502
                frame False {
                }
                frame True {
                }
              }
              n266 = Not(x=w502) -> (.not. x?=w501:bool)
              n267 = in-place-cluster #5("Unique strike parameters"=w501, "funnel state"=w505) -> (w499:T1)
            }
          }
          frame "funnel state" {
            n268 = in-place {
              n269 = in-place-cluster #6(w511) -> ("funnel state"=w514:enum16{"funnel open", "funnel closed"})  [unwired: 1 out]
              n270 = case shown="\"funnel closed\"" w514 {
                selector: w514 -> [w517 w519]
                tunnel: [w517 w519] -> w515
                tunnel: [FALSE TRUE] -> w512
                frame "funnel open", Default {
                }
                frame "funnel closed" {
                }
              }
              n271 = Not(x=w512) -> (.not. x?=w513:bool)
              n272 = in-place-cluster #6("Unique strike parameters"=w513, "funnel state"=w515) -> (w510:T1)
            }
          }
        }
        n273 = local write "scan monitor control"(w495) -> ()
      }
      event "use fast fit?": Value Change {
        n274 = event-data() -> ()  [unwired: 1 in, 6 out]
      }
      event "overwrite (d)": Value Change {
        n275 = event-data() -> ("NewVal"=w521:enum16{"DUMP", "WORK", ""})  [unwired: 1 in]
        n276 = case shown="\"DUMP\", Default" w521 {
          tunnel: [FALSE ("overwriting !!") TRUE ("overwriting !!")] -> w520
          frame "DUMP", Default {
          }
          frame "WORK" {
          }
        }
        n277 = local write "overwriting !!"(w520) -> ()
      }
      event "autopilot": Value Change {
        n278 = event-data() -> ("NewVal"=w526:enum32{"on", "off"})  [unwired: 1 in]
        n279 = local read "scan monitor control"() -> (w525:T1)
        n280 = case shown="\"on\"" w526 {
          tunnel: w525 -> [w529 w530]
          tunnel: [w527 w530] -> w524
          frame "on" {
            n281 = Bundle By Name(cluster=w529, "overwrite ctl?"=TRUE ("overwrite?")) -> (w527:T1)
          }
          frame "off", Default {
          }
        }
        n282 = local write "scan monitor control"(w524) -> ()
      }
      event "Plot: All": Cursor Move {
        n283 = event-data() -> ("CursIdx"=w531:i32)  [unwired: 1 in, 3 out]
        n284 = call "cursor window logic V2.vi"("CursIdx"=w531, "cursor window action"=cursor_window_action."cursor moves", "cursor window in"=w532) -> ()  [unwired: 7 in, 2 out]
      }
      event "Plot: All": Cursor Release {
        n285 = event-data() -> ("CursIdx"=w535:i32)  [unwired: 1 in, 3 out]
        n286 = case shown="0..2" w535 {
          tunnel: w534 -> [_ w536]
          frame 3, Default {
          }
          frame 0..2 {
            w537 = "one peak"  # event data
            n287 = Generate User Event(user event=w536, event data cluster=w537) -> ()  [unwired: 2 in, 2 out]
          }
        }
      }
      event "scale gauge: Plot: complex plane - filter": Value Change {
        n288 = event-data() -> ("NewVal"=w541:dbl)  [unwired: 1 in]
        n289 = Unbundle By Name(w539) -> ("4corners.z center"=w540:cdb)
        n290 = Unbundle By Name(w539) -> ("4corners"=→"4corners":T6)
        n291 = Complex To Re/Im(x + iy=w540) -> (x=w543:dbl, y=w544:dbl)
        n292 = Negate(x=w541) -> (-x=w549:dbl)
        n293 = control-ref of="Plot: complex plane - filter"() -> (w542:refnum<vi>)
        n294 = Add(x=w544, y=w549) -> (x+y=w545:dbl)
        n295 = Add(x=w543, y=w541) -> (x+y=w547:dbl)
        n296 = Add(x=w543, y=w549) -> (x+y=w548:dbl)
        n297 = Add(x=w544, y=w541) -> (x+y=w546:dbl)
        n298 = property on="Property Node" class="XYGraph (strict)"(reference=w542, "XScale.Minimum"=w548, "XScale.Maximum"=w547, "YScale.Maximum"=w546, "YScale.Minimum"=w545) -> ()  [unwired: 1 in, 2 out]
      }
      event "scale gauge: Plot: complex plane": Value Change {
        n299 = event-data() -> ("NewVal"=w553:dbl)  [unwired: 1 in]
        n300 = Unbundle By Name(w552) -> ("4corners.z center"=w551:cdb)
        n301 = Complex To Re/Im(x + iy=w551) -> (x=w554:dbl, y=w555:dbl)
        n302 = Negate(x=w553) -> (-x=w560:dbl)
        n303 = Add(x=w555, y=w560) -> (x+y=w556:dbl)
        n304 = Add(x=w554, y=w553) -> (x+y=w558:dbl)
        n305 = Add(x=w554, y=w560) -> (x+y=w559:dbl)
        n306 = Add(x=w555, y=w553) -> (x+y=w557:dbl)
        n307 = property on="Property Node" class="XYGraph (strict)"(reference=w550, "XScale.Minimum"=w559, "XScale.Maximum"=w558, "YScale.Maximum"=w557, "YScale.Minimum"=w556) -> ()  [unwired: 1 in, 2 out]
      }
    }
    n308 = Wait (ms)(milliseconds to wait=u32 31) -> ()  [unwired: 1 out]
  }
  n309 = control-ref of="timer \"v\""() -> (w24:refnum<vi>)
  n310 = control-ref of="timer  \"update\""() -> (w7:refnum<vi>)
  n311 = call "slider timer .vi"("action"=w6, "timer ref"=w7) -> ("timer out"=w5:refnum<vi>)  [unwired: 7 in, 2 out]
  n312 = call "slider timer .vi"("action"=w6, "timer ref"=w24) -> ("timer out"=w3:refnum<vi>)  [unwired: 7 in, 2 out]
  n313 = local read "file path"() -> (w4:path)
  n314 = call "slider timer .vi"("action"=countdown_control."stop", "timer ref"=w3) -> ("timer out"=w2:refnum<vi>)  [unwired: 7 in, 2 out]
  n315 = while {
    tunnel: w25 -> [w572]
    shift-right: [w576] -> _
    shift-left: w2 -> [w577]
    shift-right: [w570] -> _
    shift-left: w5 -> [w571]
    shift-right: [w567] -> _
    shift-left: w4 -> [w568]
    stop <- FALSE stop-if-true
    (unwired) 0
    n316 = case shown="\"on\"" "autopilot" {
      tunnel: [FALSE TRUE] -> w562
      frame "off", Default {
      }
      frame "on" {
      }
    }
    n317 = call "slider timer .vi"("action"=countdown_control."check", "timer ref"=w571) -> ("tic"=w566:bool, "timer out"=w570:refnum<vi>)  [unwired: 7 in, 1 out]
    n318 = Compound Arithmetic op=AND(w566, w562) -> (w565:bool)
    n319 = case shown="True" w565 {
      tunnel: w568 -> [w585 w589]
      tunnel: [w585 w587] -> w567
      tunnel: [FALSE w586] -> w561
      frame False {
      }
      frame True {
        n320 = local read "Sweep folder path"() -> (w594:path)
        n321 = call "latest scan file.vi"("source"=enum16{"last scan file", "manual"}."last scan file", "file path in"=w589, "sweep folder"=w594) -> ("temperature (K)"=w593:dbl, "file or folder exists?"=w588:bool, "file path out"=w590:path)  [unwired: 5 in, 1 out]
        n322 = Not Equal?(x=w590, y=w589) -> (x != y?=w591:bool)
        n323 = And(x=w588, y=w591) -> (x .and. y?=w586:bool)
        n324 = local write "Temperature (K)"(w593) -> ()
        n325 = Select(t=w590, s=w586, f=w589) -> (s? t:f=w587:path)
        n326 = local write "file path"(w587) -> ()
        n327 = local write "scan file found"(w588) -> ()
      }
    }
    n328 = Wait (ms)(milliseconds to wait=u32 123) -> ()  [unwired: 1 out]
    n329 = Select(t=countdown_control."reset once" ("action"), s=w561, f=countdown_control."check" ("action")) -> (s? t:f=w573:T16)
    n330 = call "slider timer .vi"("action"=w573, "timer ref"=w577) -> ("tic"=w564:bool, "timer out"=w576:refnum<vi>)  [unwired: 7 in, 1 out]
    n331 = And(x=w562, y=w564) -> (x .and. y?=w578:bool)
    n332 = case shown="True" w578 {
      tunnel: w572 -> [_ w595]
      frame False {
      }
      frame True {
        w596 = "scan for existing peaks"  # calculate
        n333 = Generate User Event(user event=w595, event data cluster=w596) -> ()  [unwired: 2 in, 2 out]
      }
    }
    n334 = And(x=w562, y=w561) -> (x .and. y?=w579:bool)
    n335 = case shown="True" w579 {
      tunnel: w572 -> [_ w598]
      frame False {
      }
      frame True {
        w597 = "calc:new file"  # calculate
        n336 = Generate User Event(user event=w598, event data cluster=w597) -> ()  [unwired: 2 in, 2 out]
      }
    }
  }
